vi "SMU Switch Handshaking - Debug - Continuous.vi"(8 "error in":errorcluster, 11 "file path (use dialog)":path=path "/home/lvuser/jsontestfile.json") -> (0 "error out":errorcluster)   [LabVIEW 2019]
uses:
  labview-grpc-query-server/VIs/MeasurementServer_FourProbeRawData.ctl
  labview-grpc-query-server/VIs/MeasurementServer_ErrorOutData.ctl
  JSONCluster.ctl
  <instrlib>/niDCPower/nidcpower.llb/niDCPower Send Software Edge Trigger - Signal.ctl
  <instrlib>/niDCPower/nidcpower.llb/niDCPower Wait For Event - Event.ctl
  <instrlib>/niDCPower/nidcpower.llb/niDCPower Configure Software Edge Start Trigger.vi
  <instrlib>/niDCPower/nidcpower.llb/niDCPower Configure Software Edge Sequence Advance Trigger.vi
  SupportVIs.lvlib
  labview-grpc-query-server/VIs/labview-grpc-measurement-server.lvlib
panel:
  in  "Stop":bool
  in  "Override Channel":bool
  in  "Select Next Channel":i32=39
  out "Channels Connected":string[](array[string])=["[ab0->card1r0->c39]", "[ab1->card1r1->c40]", "[ch43->com]"]
  in  "Override Settings":T1={"SMUResourceName"="SMU", "SMUChannels"="0", "SMUSourceMode"=1021, "SMUOutputFunction"=1007, "SMUSourceTransientResponse"=1038, "SMUCurrent"=1.0, "SMUCurrentLevelRange"=1.0, "SMUMeasurementSense"=1008, "SMUMeasurementApertureTime"=0.04, "SMUSourceAdvancedSourceDelay"=0.001, "SMUVoltage"=6.0, "SMUSourceAdvancedSequenceLoopCount"=162, "SMUMeasurementAdvancedDCNoiseRejection"=1044, "SMUSequenceName"="MySequence", "SMUStep1_Source_DCCurrent_CurrentLevel"=1150009, "SMUStep2_Measurement_ApertureTime"=1150058, "SMUStep3_Source_Advanced_SourceDelay"=1150051, "SMUSequenceNumberOfSteps"=3, "ScanList"="SCANALL", "Switch1ResourceName"="2526_1", "Switch1Topology"="2526/2-Wire 79x1 Mux", "Switch1ScanList"="ch70:76->com", "Switch2ResourceName"="SwitchBlock1Dev1", "Switch2Topology"="Configured Topology", "Switch2ScanList"="[c2->card1r2->c26], [c3->card1r3->c27]; [c6->card1r2->c26], [c7->card1r3->c27]; [c10->card1r2->c26], [c11->card1r3->c27]; [c14->card1r2->c26], [c15->card1r3->c27]; [c18->card1r2->c26], [c19->card1r3->c27]; [c22->card1r2->c26], [c23->card1r3->c27]; [c30->card1r2->c26], [c31->card1r3->c27];", "DMMResourceName"="DMM", "DMMFunction"=0, "DMMResolution"=0.1, "DMMRange"=0.1, "DMMSampleCount"=0, "DMMApertureTimeUnit"=0, "DMMApertureTime"=0.033, "DMMNumberOfAverages"=1, "DMMAutoZero"=0, "DMMADCCalibration"=0, "DMMSettleTime"=0.002, "DMMControlAction"=0, "DMMVoltageFaultUpperLimit"=0.0006, "ApplicationNumberOfWeldChannels"=162} {"DMMVoltageFaultUpperLimit" format="%#_6p"}
  in  "Override Settings?":bool
  out "Configured Settings":T1={"SMUResourceName"="SMU", "SMUChannels"="0", "SMUSourceMode"=1021, "SMUOutputFunction"=1007, "SMUSourceTransientResponse"=1038, "SMUCurrent"=1.0, "SMUCurrentLevelRange"=1.0, "SMUMeasurementSense"=1008, "SMUMeasurementApertureTime"=0.04, "SMUSourceAdvancedSourceDelay"=0.001, "SMUVoltage"=6.0, "SMUSourceAdvancedSequenceLoopCount"=162, "SMUMeasurementAdvancedDCNoiseRejection"=1044, "SMUSequenceName"="MySequence", "SMUStep1_Source_DCCurrent_CurrentLevel"=1150009, "SMUStep2_Measurement_ApertureTime"=1150058, "SMUStep3_Source_Advanced_SourceDelay"=1150051, "SMUSequenceNumberOfSteps"=3, "ScanList"="SCANALL", "Switch1ResourceName"="2526_1", "Switch1Topology"="2526/2-Wire 79x1 Mux", "Switch1ScanList"="ch70:76->com", "Switch2ResourceName"="SwitchBlock1Dev1", "Switch2Topology"="Configured Topology", "Switch2ScanList"="[c2->card1r2->c26], [c3->card1r3->c27]; [c6->card1r2->c26], [c7->card1r3->c27]; [c10->card1r2->c26], [c11->card1r3->c27]; [c14->card1r2->c26], [c15->card1r3->c27]; [c18->card1r2->c26], [c19->card1r3->c27]; [c22->card1r2->c26], [c23->card1r3->c27]; [c30->card1r2->c26], [c31->card1r3->c27];", "DMMResourceName"="DMM", "DMMFunction"=0, "DMMResolution"=0.1, "DMMRange"=0.1, "DMMSampleCount"=0, "DMMApertureTimeUnit"=0, "DMMApertureTime"=0.033, "DMMNumberOfAverages"=1, "DMMAutoZero"=0, "DMMADCCalibration"=0, "DMMSettleTime"=0.002, "DMMControlAction"=0, "DMMVoltageFaultUpperLimit"=0.0006, "ApplicationNumberOfWeldChannels"=162} {"DMMVoltageFaultUpperLimit" format="%#_6p"}
  out "All Results":T2[](array[typedef])=[{"Positive Voltage"=-0.05653296298856869, "Positive Current"=2.9701845245998226e-05, "Negative Voltage"=nan, "Negative Current"=3.073839441384771e-05, "Impedance"=nan, "ErrorOutData"={"ErrorCode"=-3, "ErrorMessage"="SMU HI or LO lead disconnected\n- SMU in compliance\n- SMU Fault = True\rDMM HI SENSE or LO SENSE lead disconnected\n- DMM measures NaN, or \n- DMM overrange warning, or\n- DMM voltage > 50uV "}}, {"Positive Voltage"=nan, "Positive Current"=2.9670434665157036e-05, "Negative Voltage"=nan, "Negative Current"=3.076980499469237e-05, "Impedance"=nan, "ErrorOutData"={"ErrorCode"=-3, "ErrorMessage"="SMU HI or LO lead disconnected\n- SMU in compliance\n- SMU Fault = True\rDMM HI SENSE or LO SENSE lead disconnected\n- DMM measures NaN, or \n- DMM overrange warning, or\n- DMM voltage > 50uV "}}, {"Positive Voltage"=nan, "Positive Current"=2.9796076988532205e-05, "Negative Voltage"=nan, "Negative Current"=3.070698383300305e-05, "Impedance"=nan, "ErrorOutData"={"ErrorCode"=-3, "ErrorMessage"="SMU HI or LO lead disconnected\n- SMU in compliance\n- SMU Fault = True\rDMM HI SENSE or LO SENSE lead disconnected\n- DMM measures NaN, or \n- DMM overrange warning, or\n- DMM voltage > 50uV "}}, {"Positive Voltage"=nan, "Positive Current"=2.9921719311907374e-05, "Negative Voltage"=nan, "Negative Current"=3.083262615638169e-05, "Impedance"=nan, "ErrorOutData"={"ErrorCode"=-3, "ErrorMessage"="SMU HI or LO lead disconnected\n- SMU in compliance\n- SMU Fault = True\rDMM HI SENSE or LO SENSE lead disconnected\n- DMM measures NaN, or \n- DMM overrange warning, or\n- DMM voltage > 50uV "}}, {"Positive Voltage"=nan, "Positive Current"=2.9796076988532205e-05, "Negative Voltage"=-0.04961459275744348, "Negative Current"=3.06441626713172e-05, "Impedance"=nan, "ErrorOutData"={"ErrorCode"=-3, "ErrorMessage"="SMU HI or LO lead disconnected\n- SMU in compliance\n- SMU Fault = True\rDMM HI SENSE or LO SENSE lead disconnected\n- DMM measures NaN, or \n- DMM overrange warning, or\n- DMM voltage > 50uV "}}, {"Positive Voltage"=nan, "Positive Current"=2.9858898150218055e-05, "Negative Voltage"=-0.05577502096881172, "Negative Current"=3.080121557553703e-05, "Impedance"=nan, "ErrorOutData"={"ErrorCode"=-3, "ErrorMessage"="SMU HI or LO lead disconnected\n- SMU in compliance\n- SMU Fault = True\rDMM HI SENSE or LO SENSE lead disconnected\n- DMM measures NaN, or \n- DMM overrange warning, or\n- DMM voltage > 50uV "}}, {"Positive Voltage"=0.02445423618825113, "Positive Current"=2.9890308731062715e-05, "Negative Voltage"=nan, "Negative Current"=3.09268578989122e-05, "Impedance"=nan, "ErrorOutData"={"ErrorCode"=-3, "ErrorMessage"="SMU HI or LO lead disconnected\n- SMU in compliance\n- SMU Fault = True\rDMM HI SENSE or LO SENSE lead disconnected\n- DMM measures NaN, or \n- DMM overrange warning, or\n- DMM voltage > 50uV "}}, {"Positive Voltage"=nan, "Positive Current"=2.9639024084312376e-05, "Negative Voltage"=0.01690976674095387, "Negative Current"=3.086403673722288e-05, "Impedance"=nan, "ErrorOutData"={"ErrorCode"=-3, "ErrorMessage"="SMU HI or LO lead disconnected\n- SMU in compliance\n- SMU Fault = True\rDMM HI SENSE or LO SENSE lead disconnected\n- DMM measures NaN, or \n- DMM overrange warning, or\n- DMM voltage > 50uV "}}, {"Positive Voltage"=nan, "Positive Current"=1.0000000232887618, "Negative Voltage"=-0.02788016487004771, "Negative Current"=-0.999999922774903, "Impedance"=nan, "ErrorOutData"={"ErrorCode"=-2, "ErrorMessage"="\rDMM HI SENSE or LO SENSE lead disconnected\n- DMM measures NaN, or \n- DMM overrange warning, or\n- DMM voltage > 50uV "}}, {"Positive Voltage"=nan, "Positive Current"=2.9764666407687546e-05, "Negative Voltage"=nan, "Negative Current"=3.076980499469237e-05, "Impedance"=nan, "ErrorOutData"={"ErrorCode"=-3, "ErrorMessage"="SMU HI or LO lead disconnected\n- SMU in compliance\n- SMU Fault = True\rDMM HI SENSE or LO SENSE lead disconnected\n- DMM measures NaN, or \n- DMM overrange warning, or\n- DMM voltage > 50uV "}}, {"Positive Voltage"=nan, "Positive Current"=2.9733255826842886e-05, "Negative Voltage"=nan, "Negative Current"=3.080121557553703e-05, "Impedance"=nan, "ErrorOutData"={"ErrorCode"=-3, "ErrorMessage"="SMU HI or LO lead disconnected\n- SMU in compliance\n- SMU Fault = True\rDMM HI SENSE or LO SENSE lead disconnected\n- DMM measures NaN, or \n- DMM overrange warning, or\n- DMM voltage > 50uV "}}, {"Positive Voltage"=nan, "Positive Current"=2.9764666407687546e-05, "Negative Voltage"=nan, "Negative Current"=3.070698383300305e-05, "Impedance"=nan, "ErrorOutData"={"ErrorCode"=-3, "ErrorMessage"="SMU HI or LO lead disconnected\n- SMU in compliance\n- SMU Fault = True\rDMM HI SENSE or LO SENSE lead disconnected\n- DMM measures NaN, or \n- DMM overrange warning, or\n- DMM voltage > 50uV "}}, {"Positive Voltage"=nan, "Positive Current"=2.9858898150218055e-05, "Negative Voltage"=-0.032372464954530354, "Negative Current"=3.073839441384771e-05, "Impedance"=nan, "ErrorOutData"={"ErrorCode"=-3, "ErrorMessage"="SMU HI or LO lead disconnected\n- SMU in compliance\n- SMU Fault = True\rDMM HI SENSE or LO SENSE lead disconnected\n- DMM measures NaN, or \n- DMM overrange warning, or\n- DMM voltage > 50uV "}}, {"Positive Voltage"=nan, "Positive Current"=2.9921719311907374e-05, "Negative Voltage"=nan, "Negative Current"=3.09268578989122e-05, "Impedance"=nan, "ErrorOutData"={"ErrorCode"=-3, "ErrorMessage"="SMU HI or LO lead disconnected\n- SMU in compliance\n- SMU Fault = True\rDMM HI SENSE or LO SENSE lead disconnected\n- DMM measures NaN, or \n- DMM overrange warning, or\n- DMM voltage > 50uV "}}, {"Positive Voltage"=nan, "Positive Current"=2.9858898150218055e-05, "Negative Voltage"=nan, "Negative Current"=3.0958268479756856e-05, "Impedance"=nan, "ErrorOutData"={"ErrorCode"=-3, "ErrorMessage"="SMU HI or LO lead disconnected\n- SMU in compliance\n- SMU Fault = True\rDMM HI SENSE or LO SENSE lead disconnected\n- DMM measures NaN, or \n- DMM overrange warning, or\n- DMM voltage > 50uV "}}, {"Positive Voltage"=nan, "Positive Current"=2.9764666407687546e-05, "Negative Voltage"=-0.05143121180189266, "Negative Current"=3.067557325216186e-05, "Impedance"=nan, "ErrorOutData"={"ErrorCode"=-3, "ErrorMessage"="SMU HI or LO lead disconnected\n- SMU in compliance\n- SMU Fault = True\rDMM HI SENSE or LO SENSE lead disconnected\n- DMM measures NaN, or \n- DMM overrange warning, or\n- DMM voltage > 50uV "}}, {"Positive Voltage"=nan, "Positive Current"=2.9921719311907374e-05, "Negative Voltage"=nan, "Negative Current"=3.073839441384771e-05, "Impedance"=nan, "ErrorOutData"={"ErrorCode"=-3, "ErrorMessage"="SMU HI or LO lead disconnected\n- SMU in compliance\n- SMU Fault = True\rDMM HI SENSE or LO SENSE lead disconnected\n- DMM measures NaN, or \n- DMM overrange warning, or\n- DMM voltage > 50uV "}}, {"Positive Voltage"=nan, "Positive Current"=2.9796076988532205e-05, "Negative Voltage"=nan, "Negative Current"=3.080121557553703e-05, "Impedance"=nan, "ErrorOutData"={"ErrorCode"=-3, "ErrorMessage"="SMU HI or LO lead disconnected\n- SMU in compliance\n- SMU Fault = True\rDMM HI SENSE or LO SENSE lead disconnected\n- DMM measures NaN, or \n- DMM overrange warning, or\n- DMM voltage > 50uV "}}, {"Positive Voltage"=nan, "Positive Current"=2.9764666407687546e-05, "Negative Voltage"=nan, "Negative Current"=3.089544731806754e-05, "Impedance"=nan, "ErrorOutData"={"ErrorCode"=-3, "ErrorMessage"="SMU HI or LO lead disconnected\n- SMU in compliance\n- SMU Fault = True\rDMM HI SENSE or LO SENSE lead disconnected\n- DMM measures NaN, or \n- DMM overrange warning, or\n- DMM voltage > 50uV "}}, {"Positive Voltage"=nan, "Positive Current"=2.9796076988532205e-05, "Negative Voltage"=nan, "Negative Current"=3.067557325216186e-05, "Impedance"=nan, "ErrorOutData"={"ErrorCode"=-3, "ErrorMessage"="SMU HI or LO lead disconnected\n- SMU in compliance\n- SMU Fault = True\rDMM HI SENSE or LO SENSE lead disconnected\n- DMM measures NaN, or \n- DMM overrange warning, or\n- DMM voltage > 50uV "}}, {"Positive Voltage"=nan, "Positive Current"=2.9827487569376865e-05, "Negative Voltage"=nan, "Negative Current"=3.058134150963135e-05, "Impedance"=nan, "ErrorOutData"={"ErrorCode"=-3, "ErrorMessage"="SMU HI or LO lead disconnected\n- SMU in compliance\n- SMU Fault = True\rDMM HI SENSE or LO SENSE lead disconnected\n- DMM measures NaN, or \n- DMM overrange warning, or\n- DMM voltage > 50uV "}}, {"Positive Voltage"=0.0611653266410722, "Positive Current"=2.9701845245998226e-05, "Negative Voltage"=nan, "Negative Current"=3.058134150963135e-05, "Impedance"=nan, "ErrorOutData"={"ErrorCode"=-3, "ErrorMessage"="SMU HI or LO lead disconnected\n- SMU in compliance\n- SMU Fault = True\rDMM HI SENSE or LO SENSE lead disconnected\n- DMM measures NaN, or \n- DMM overrange warning, or\n- DMM voltage > 50uV "}}, {"Positive Voltage"=nan, "Positive Current"=2.9607613503467717e-05, "Negative Voltage"=nan, "Negative Current"=3.086403673722288e-05, "Impedance"=nan, "ErrorOutData"={"ErrorCode"=-3, "ErrorMessage"="SMU HI or LO lead disconnected\n- SMU in compliance\n- SMU Fault = True\rDMM HI SENSE or LO SENSE lead disconnected\n- DMM measures NaN, or \n- DMM overrange warning, or\n- DMM voltage > 50uV "}}, {"Positive Voltage"=nan, "Positive Current"=2.9796076988532205e-05, "Negative Voltage"=nan, "Negative Current"=3.086403673722288e-05, "Impedance"=nan, "ErrorOutData"={"ErrorCode"=-3, "ErrorMessage"="SMU HI or LO lead disconnected\n- SMU in compliance\n- SMU Fault = True\rDMM HI SENSE or LO SENSE lead disconnected\n- DMM measures NaN, or \n- DMM overrange warning, or\n- DMM voltage > 50uV "}}, {"Positive Voltage"=nan, "Positive Current"=2.9670434665157036e-05, "Negative Voltage"=nan, "Negative Current"=3.06441626713172e-05, "Impedance"=nan, "ErrorOutData"={"ErrorCode"=-3, "ErrorMessage"="SMU HI or LO lead disconnected\n- SMU in compliance\n- SMU Fault = True\rDMM HI SENSE or LO SENSE lead disconnected\n- DMM measures NaN, or \n- DMM overrange warning, or\n- DMM voltage > 50uV "}}, {"Positive Voltage"=nan, "Positive Current"=2.9858898150218055e-05, "Negative Voltage"=nan, "Negative Current"=3.067557325216186e-05, "Impedance"=nan, "ErrorOutData"={"ErrorCode"=-3, "ErrorMessage"="SMU HI or LO lead disconnected\n- SMU in compliance\n- SMU Fault = True\rDMM HI SENSE or LO SENSE lead disconnected\n- DMM measures NaN, or \n- DMM overrange warning, or\n- DMM voltage > 50uV "}}, {"Positive Voltage"=nan, "Positive Current"=2.9890308731062715e-05, "Negative Voltage"=nan, "Negative Current"=3.080121557553703e-05, "Impedance"=nan, "ErrorOutData"={"ErrorCode"=-3, "ErrorMessage"="SMU HI or LO lead disconnected\n- SMU in compliance\n- SMU Fault = True\rDMM HI SENSE or LO SENSE lead disconnected\n- DMM measures NaN, or \n- DMM overrange warning, or\n- DMM voltage > 50uV "}}, {"Positive Voltage"=nan, "Positive Current"=2.9733255826842886e-05, "Negative Voltage"=nan, "Negative Current"=3.073839441384771e-05, "Impedance"=nan, "ErrorOutData"={"ErrorCode"=-3, "ErrorMessage"="SMU HI or LO lead disconnected\n- SMU in compliance\n- SMU Fault = True\rDMM HI SENSE or LO SENSE lead disconnected\n- DMM measures NaN, or \n- DMM overrange warning, or\n- DMM voltage > 50uV "}}, {"Positive Voltage"=nan, "Positive Current"=2.9670434665157036e-05, "Negative Voltage"=-0.05787915599385992, "Negative Current"=3.073839441384771e-05, "Impedance"=nan, "ErrorOutData"={"ErrorCode"=-3, "ErrorMessage"="SMU HI or LO lead disconnected\n- SMU in compliance\n- SMU Fault = True\rDMM HI SENSE or LO SENSE lead disconnected\n- DMM measures NaN, or \n- DMM overrange warning, or\n- DMM voltage > 50uV "}}, {"Positive Voltage"=nan, "Positive Current"=2.9639024084312376e-05, "Negative Voltage"=nan, "Negative Current"=3.058134150963135e-05, "Impedance"=nan, "ErrorOutData"={"ErrorCode"=-3, "ErrorMessage"="SMU HI or LO lead disconnected\n- SMU in compliance\n- SMU Fault = True\rDMM HI SENSE or LO SENSE lead disconnected\n- DMM measures NaN, or \n- DMM overrange warning, or\n- DMM voltage > 50uV "}}, {"Positive Voltage"=nan, "Positive Current"=2.9513381760937207e-05, "Negative Voltage"=nan, "Negative Current"=3.054993092878322e-05, "Impedance"=nan, "ErrorOutData"={"ErrorCode"=-3, "ErrorMessage"="SMU HI or LO lead disconnected\n- SMU in compliance\n- SMU Fault = True\rDMM HI SENSE or LO SENSE lead disconnected\n- DMM measures NaN, or \n- DMM overrange warning, or\n- DMM voltage > 50uV "}}, {"Positive Voltage"=nan, "Positive Current"=2.9670434665157036e-05, "Negative Voltage"=nan, "Negative Current"=3.061275209047254e-05, "Impedance"=nan, "ErrorOutData"={"ErrorCode"=-3, "ErrorMessage"="SMU HI or LO lead disconnected\n- SMU in compliance\n- SMU Fault = True\rDMM HI SENSE or LO SENSE lead disconnected\n- DMM measures NaN, or \n- DMM overrange warning, or\n- DMM voltage > 50uV "}}, {"Positive Voltage"=nan, "Positive Current"=2.9701845245998226e-05, "Negative Voltage"=nan, "Negative Current"=3.061275209047254e-05, "Impedance"=nan, "ErrorOutData"={"ErrorCode"=-3, "ErrorMessage"="SMU HI or LO lead disconnected\n- SMU in compliance\n- SMU Fault = True\rDMM HI SENSE or LO SENSE lead disconnected\n- DMM measures NaN, or \n- DMM overrange warning, or\n- DMM voltage > 50uV "}}, {"Positive Voltage"=nan, "Positive Current"=2.9544792341781867e-05, "Negative Voltage"=nan, "Negative Current"=3.067557325216186e-05, "Impedance"=nan, "ErrorOutData"={"ErrorCode"=-3, "ErrorMessage"="SMU HI or LO lead disconnected\n- SMU in compliance\n- SMU Fault = True\rDMM HI SENSE or LO SENSE lead disconnected\n- DMM measures NaN, or \n- DMM overrange warning, or\n- DMM voltage > 50uV "}}, {"Positive Voltage"=nan, "Positive Current"=2.9701845245998226e-05, "Negative Voltage"=nan, "Negative Current"=3.073839441384771e-05, "Impedance"=nan, "ErrorOutData"={"ErrorCode"=-3, "ErrorMessage"="SMU HI or LO lead disconnected\n- SMU in compliance\n- SMU Fault = True\rDMM HI SENSE or LO SENSE lead disconnected\n- DMM measures NaN, or \n- DMM overrange warning, or\n- DMM voltage > 50uV "}}, {"Positive Voltage"=nan, "Positive Current"=2.9513381760937207e-05, "Negative Voltage"=nan, "Negative Current"=3.06441626713172e-05, "Impedance"=nan, "ErrorOutData"={"ErrorCode"=-3, "ErrorMessage"="SMU HI or LO lead disconnected\n- SMU in compliance\n- SMU Fault = True\rDMM HI SENSE or LO SENSE lead disconnected\n- DMM measures NaN, or \n- DMM overrange warning, or\n- DMM voltage > 50uV "}}, {"Positive Voltage"=nan, "Positive Current"=2.9576202922623057e-05, "Negative Voltage"=0.0032061164902873482, "Negative Current"=3.070698383300305e-05, "Impedance"=nan, "ErrorOutData"={"ErrorCode"=-3, "ErrorMessage"="SMU HI or LO lead disconnected\n- SMU in compliance\n- SMU Fault = True\rDMM HI SENSE or LO SENSE lead disconnected\n- DMM measures NaN, or \n- DMM overrange warning, or\n- DMM voltage > 50uV "}}, {"Positive Voltage"=nan, "Positive Current"=2.9607613503467717e-05, "Negative Voltage"=-0.0014952361703153266, "Negative Current"=3.083262615638169e-05, "Impedance"=nan, "ErrorOutData"={"ErrorCode"=-3, "ErrorMessage"="SMU HI or LO lead disconnected\n- SMU in compliance\n- SMU Fault = True\rDMM HI SENSE or LO SENSE lead disconnected\n- DMM measures NaN, or \n- DMM overrange warning, or\n- DMM voltage > 50uV "}}, {"Positive Voltage"=nan, "Positive Current"=2.9796076988532205e-05, "Negative Voltage"=0.02077001908732105, "Negative Current"=3.080121557553703e-05, "Impedance"=nan, "ErrorOutData"={"ErrorCode"=-3, "ErrorMessage"="SMU HI or LO lead disconnected\n- SMU in compliance\n- SMU Fault = True\rDMM HI SENSE or LO SENSE lead disconnected\n- DMM measures NaN, or \n- DMM overrange warning, or\n- DMM voltage > 50uV "}}, {"Positive Voltage"=nan, "Positive Current"=2.9670434665157036e-05, "Negative Voltage"=0.030919103420959628, "Negative Current"=3.083262615638169e-05, "Impedance"=nan, "ErrorOutData"={"ErrorCode"=-3, "ErrorMessage"="SMU HI or LO lead disconnected\n- SMU in compliance\n- SMU Fault = True\rDMM HI SENSE or LO SENSE lead disconnected\n- DMM measures NaN, or \n- DMM overrange warning, or\n- DMM voltage > 50uV "}}, {"Positive Voltage"=nan, "Positive Current"=1.000000965606187, "Negative Voltage"=-0.057247959131579734, "Negative Current"=-1.0000000170066456, "Impedance"=nan, "ErrorOutData"={"ErrorCode"=-2, "ErrorMessage"="\rDMM HI SENSE or LO SENSE lead disconnected\n- DMM measures NaN, or \n- DMM overrange warning, or\n- DMM voltage > 50uV "}}, {"Positive Voltage"=nan, "Positive Current"=2.9576202922623057e-05, "Negative Voltage"=nan, "Negative Current"=3.06441626713172e-05, "Impedance"=nan, "ErrorOutData"={"ErrorCode"=-3, "ErrorMessage"="SMU HI or LO lead disconnected\n- SMU in compliance\n- SMU Fault = True\rDMM HI SENSE or LO SENSE lead disconnected\n- DMM measures NaN, or \n- DMM overrange warning, or\n- DMM voltage > 50uV "}}, {"Positive Voltage"=nan, "Positive Current"=2.9544792341781867e-05, "Negative Voltage"=nan, "Negative Current"=3.067557325216186e-05, "Impedance"=nan, "ErrorOutData"={"ErrorCode"=-3, "ErrorMessage"="SMU HI or LO lead disconnected\n- SMU in compliance\n- SMU Fault = True\rDMM HI SENSE or LO SENSE lead disconnected\n- DMM measures NaN, or \n- DMM overrange warning, or\n- DMM voltage > 50uV "}}, {"Positive Voltage"=nan, "Positive Current"=2.9764666407687546e-05, "Negative Voltage"=nan, "Negative Current"=3.073839441384771e-05, "Impedance"=nan, "ErrorOutData"={"ErrorCode"=-3, "ErrorMessage"="SMU HI or LO lead disconnected\n- SMU in compliance\n- SMU Fault = True\rDMM HI SENSE or LO SENSE lead disconnected\n- DMM measures NaN, or \n- DMM overrange warning, or\n- DMM voltage > 50uV "}}, {"Positive Voltage"=0.034574482900608876, "Positive Current"=2.9576202922623057e-05, "Negative Voltage"=nan, "Negative Current"=3.054993092878322e-05, "Impedance"=nan, "ErrorOutData"={"ErrorCode"=-3, "ErrorMessage"="SMU HI or LO lead disconnected\n- SMU in compliance\n- SMU Fault = True\rDMM HI SENSE or LO SENSE lead disconnected\n- DMM measures NaN, or \n- DMM overrange warning, or\n- DMM voltage > 50uV "}}, {"Positive Voltage"=nan, "Positive Current"=2.9639024084312376e-05, "Negative Voltage"=nan, "Negative Current"=3.048710976709737e-05, "Impedance"=nan, "ErrorOutData"={"ErrorCode"=-3, "ErrorMessage"="SMU HI or LO lead disconnected\n- SMU in compliance\n- SMU Fault = True\rDMM HI SENSE or LO SENSE lead disconnected\n- DMM measures NaN, or \n- DMM overrange warning, or\n- DMM voltage > 50uV "}}, {"Positive Voltage"=nan, "Positive Current"=2.9481971180092548e-05, "Negative Voltage"=nan, "Negative Current"=3.033005686287754e-05, "Impedance"=nan, "ErrorOutData"={"ErrorCode"=-3, "ErrorMessage"="SMU HI or LO lead disconnected\n- SMU in compliance\n- SMU Fault = True\rDMM HI SENSE or LO SENSE lead disconnected\n- DMM measures NaN, or \n- DMM overrange warning, or\n- DMM voltage > 50uV "}}, {"Positive Voltage"=nan, "Positive Current"=2.9387739437562038e-05, "Negative Voltage"=nan, "Negative Current"=3.03614674437222e-05, "Impedance"=nan, "ErrorOutData"={"ErrorCode"=-3, "ErrorMessage"="SMU HI or LO lead disconnected\n- SMU in compliance\n- SMU Fault = True\rDMM HI SENSE or LO SENSE lead disconnected\n- DMM measures NaN, or \n- DMM overrange warning, or\n- DMM voltage > 50uV "}}, {"Positive Voltage"=nan, "Positive Current"=2.941915001840323e-05, "Negative Voltage"=nan, "Negative Current"=3.029864628203288e-05, "Impedance"=nan, "ErrorOutData"={"ErrorCode"=-3, "ErrorMessage"="SMU HI or LO lead disconnected\n- SMU in compliance\n- SMU Fault = True\rDMM HI SENSE or LO SENSE lead disconnected\n- DMM measures NaN, or \n- DMM overrange warning, or\n- DMM voltage > 50uV "}}, {"Positive Voltage"=-0.0212574588174508, "Positive Current"=2.9387739437562038e-05, "Negative Voltage"=nan, "Negative Current"=3.03614674437222e-05, "Impedance"=nan, "ErrorOutData"={"ErrorCode"=-3, "ErrorMessage"="SMU HI or LO lead disconnected\n- SMU in compliance\n- SMU Fault = True\rDMM HI SENSE or LO SENSE lead disconnected\n- DMM measures NaN, or \n- DMM overrange warning, or\n- DMM voltage > 50uV "}}, {"Positive Voltage"=nan, "Positive Current"=2.929350769502806e-05, "Negative Voltage"=nan, "Negative Current"=3.0267235701188222e-05, "Impedance"=nan, "ErrorOutData"={"ErrorCode"=-3, "ErrorMessage"="SMU HI or LO lead disconnected\n- SMU in compliance\n- SMU Fault = True\rDMM HI SENSE or LO SENSE lead disconnected\n- DMM measures NaN, or \n- DMM overrange warning, or\n- DMM voltage > 50uV "}}, {"Positive Voltage"=nan, "Positive Current"=2.9450560599247888e-05, "Negative Voltage"=nan, "Negative Current"=3.0173003958657713e-05, "Impedance"=nan, "ErrorOutData"={"ErrorCode"=-3, "ErrorMessage"="SMU HI or LO lead disconnected\n- SMU in compliance\n- SMU Fault = True\rDMM HI SENSE or LO SENSE lead disconnected\n- DMM measures NaN, or \n- DMM overrange warning, or\n- DMM voltage > 50uV "}}, {"Positive Voltage"=0.03294451244138388, "Positive Current"=2.9576202922623057e-05, "Negative Voltage"=-0.06000793949129106, "Negative Current"=3.0204414539502372e-05, "Impedance"=-147963.59926360915, "ErrorOutData"={"ErrorCode"=-3, "ErrorMessage"="SMU HI or LO lead disconnected\n- SMU in compliance\n- SMU Fault = True\rDMM HI SENSE or LO SENSE lead disconnected\n- DMM measures NaN, or \n- DMM overrange warning, or\n- DMM voltage > 50uV "}}, {"Positive Voltage"=nan, "Positive Current"=2.935632885671738e-05, "Negative Voltage"=nan, "Negative Current"=3.03614674437222e-05, "Impedance"=nan, "ErrorOutData"={"ErrorCode"=-3, "ErrorMessage"="SMU HI or LO lead disconnected\n- SMU in compliance\n- SMU Fault = True\rDMM HI SENSE or LO SENSE lead disconnected\n- DMM measures NaN, or \n- DMM overrange warning, or\n- DMM voltage > 50uV "}}, {"Positive Voltage"=nan, "Positive Current"=2.9576202922623057e-05, "Negative Voltage"=nan, "Negative Current"=3.045569918625271e-05, "Impedance"=nan, "ErrorOutData"={"ErrorCode"=-3, "ErrorMessage"="SMU HI or LO lead disconnected\n- SMU in compliance\n- SMU Fault = True\rDMM HI SENSE or LO SENSE lead disconnected\n- DMM measures NaN, or \n- DMM overrange warning, or\n- DMM voltage > 50uV "}}, {"Positive Voltage"=nan, "Positive Current"=2.941915001840323e-05, "Negative Voltage"=nan, "Negative Current"=3.058134150963135e-05, "Impedance"=nan, "ErrorOutData"={"ErrorCode"=-3, "ErrorMessage"="SMU HI or LO lead disconnected\n- SMU in compliance\n- SMU Fault = True\rDMM HI SENSE or LO SENSE lead disconnected\n- DMM measures NaN, or \n- DMM overrange warning, or\n- DMM voltage > 50uV "}}, {"Positive Voltage"=nan, "Positive Current"=2.935632885671738e-05, "Negative Voltage"=nan, "Negative Current"=3.048710976709737e-05, "Impedance"=nan, "ErrorOutData"={"ErrorCode"=-3, "ErrorMessage"="SMU HI or LO lead disconnected\n- SMU in compliance\n- SMU Fault = True\rDMM HI SENSE or LO SENSE lead disconnected\n- DMM measures NaN, or \n- DMM overrange warning, or\n- DMM voltage > 50uV "}}, {"Positive Voltage"=nan, "Positive Current"=2.9481971180092548e-05, "Negative Voltage"=nan, "Negative Current"=3.042428860541152e-05, "Impedance"=nan, "ErrorOutData"={"ErrorCode"=-3, "ErrorMessage"="SMU HI or LO lead disconnected\n- SMU in compliance\n- SMU Fault = True\rDMM HI SENSE or LO SENSE lead disconnected\n- DMM measures NaN, or \n- DMM overrange warning, or\n- DMM voltage > 50uV "}}, {"Positive Voltage"=nan, "Positive Current"=2.9576202922623057e-05, "Negative Voltage"=nan, "Negative Current"=3.058134150963135e-05, "Impedance"=nan, "ErrorOutData"={"ErrorCode"=-3, "ErrorMessage"="SMU HI or LO lead disconnected\n- SMU in compliance\n- SMU Fault = True\rDMM HI SENSE or LO SENSE lead disconnected\n- DMM measures NaN, or \n- DMM overrange warning, or\n- DMM voltage > 50uV "}}, {"Positive Voltage"=nan, "Positive Current"=2.9796076988532205e-05, "Negative Voltage"=nan, "Negative Current"=3.061275209047254e-05, "Impedance"=nan, "ErrorOutData"={"ErrorCode"=-3, "ErrorMessage"="SMU HI or LO lead disconnected\n- SMU in compliance\n- SMU Fault = True\rDMM HI SENSE or LO SENSE lead disconnected\n- DMM measures NaN, or \n- DMM overrange warning, or\n- DMM voltage > 50uV "}}, {"Positive Voltage"=nan, "Positive Current"=2.9701845245998226e-05, "Negative Voltage"=nan, "Negative Current"=3.06441626713172e-05, "Impedance"=nan, "ErrorOutData"={"ErrorCode"=-3, "ErrorMessage"="SMU HI or LO lead disconnected\n- SMU in compliance\n- SMU Fault = True\rDMM HI SENSE or LO SENSE lead disconnected\n- DMM measures NaN, or \n- DMM overrange warning, or\n- DMM voltage > 50uV "}}, {"Positive Voltage"=nan, "Positive Current"=2.9701845245998226e-05, "Negative Voltage"=nan, "Negative Current"=3.076980499469237e-05, "Impedance"=nan, "ErrorOutData"={"ErrorCode"=-3, "ErrorMessage"="SMU HI or LO lead disconnected\n- SMU in compliance\n- SMU Fault = True\rDMM HI SENSE or LO SENSE lead disconnected\n- DMM measures NaN, or \n- DMM overrange warning, or\n- DMM voltage > 50uV "}}, {"Positive Voltage"=nan, "Positive Current"=2.9544792341781867e-05, "Negative Voltage"=nan, "Negative Current"=3.042428860541152e-05, "Impedance"=nan, "ErrorOutData"={"ErrorCode"=-3, "ErrorMessage"="SMU HI or LO lead disconnected\n- SMU in compliance\n- SMU Fault = True\rDMM HI SENSE or LO SENSE lead disconnected\n- DMM measures NaN, or \n- DMM overrange warning, or\n- DMM voltage > 50uV "}}, {"Positive Voltage"=nan, "Positive Current"=2.9639024084312376e-05, "Negative Voltage"=nan, "Negative Current"=3.058134150963135e-05, "Impedance"=nan, "ErrorOutData"={"ErrorCode"=-3, "ErrorMessage"="SMU HI or LO lead disconnected\n- SMU in compliance\n- SMU Fault = True\rDMM HI SENSE or LO SENSE lead disconnected\n- DMM measures NaN, or \n- DMM overrange warning, or\n- DMM voltage > 50uV "}}, {"Positive Voltage"=nan, "Positive Current"=2.9796076988532205e-05, "Negative Voltage"=nan, "Negative Current"=3.070698383300305e-05, "Impedance"=nan, "ErrorOutData"={"ErrorCode"=-3, "ErrorMessage"="SMU HI or LO lead disconnected\n- SMU in compliance\n- SMU Fault = True\rDMM HI SENSE or LO SENSE lead disconnected\n- DMM measures NaN, or \n- DMM overrange warning, or\n- DMM voltage > 50uV "}}, {"Positive Voltage"=nan, "Positive Current"=2.9607613503467717e-05, "Negative Voltage"=nan, "Negative Current"=3.06441626713172e-05, "Impedance"=nan, "ErrorOutData"={"ErrorCode"=-3, "ErrorMessage"="SMU HI or LO lead disconnected\n- SMU in compliance\n- SMU Fault = True\rDMM HI SENSE or LO SENSE lead disconnected\n- DMM measures NaN, or \n- DMM overrange warning, or\n- DMM voltage > 50uV "}}, {"Positive Voltage"=nan, "Positive Current"=2.9576202922623057e-05, "Negative Voltage"=nan, "Negative Current"=3.06441626713172e-05, "Impedance"=nan, "ErrorOutData"={"ErrorCode"=-3, "ErrorMessage"="SMU HI or LO lead disconnected\n- SMU in compliance\n- SMU Fault = True\rDMM HI SENSE or LO SENSE lead disconnected\n- DMM measures NaN, or \n- DMM overrange warning, or\n- DMM voltage > 50uV "}}, {"Positive Voltage"=nan, "Positive Current"=2.9513381760937207e-05, "Negative Voltage"=nan, "Negative Current"=3.058134150963135e-05, "Impedance"=nan, "ErrorOutData"={"ErrorCode"=-3, "ErrorMessage"="SMU HI or LO lead disconnected\n- SMU in compliance\n- SMU Fault = True\rDMM HI SENSE or LO SENSE lead disconnected\n- DMM measures NaN, or \n- DMM overrange warning, or\n- DMM voltage > 50uV "}}, {"Positive Voltage"=nan, "Positive Current"=2.9576202922623057e-05, "Negative Voltage"=nan, "Negative Current"=3.051852034794203e-05, "Impedance"=nan, "ErrorOutData"={"ErrorCode"=-3, "ErrorMessage"="SMU HI or LO lead disconnected\n- SMU in compliance\n- SMU Fault = True\rDMM HI SENSE or LO SENSE lead disconnected\n- DMM measures NaN, or \n- DMM overrange warning, or\n- DMM voltage > 50uV "}}, {"Positive Voltage"=-0.0305689879447921, "Positive Current"=2.9670434665157036e-05, "Negative Voltage"=0.035390038606321006, "Negative Current"=3.067557325216186e-05, "Impedance"=65621.82310367978, "ErrorOutData"={"ErrorCode"=-1, "ErrorMessage"="SMU HI or LO lead disconnected\n- SMU in compliance\n- SMU Fault = True\r"}}, {"Positive Voltage"=nan, "Positive Current"=2.9701845245998226e-05, "Negative Voltage"=nan, "Negative Current"=3.042428860541152e-05, "Impedance"=nan, "ErrorOutData"={"ErrorCode"=-3, "ErrorMessage"="SMU HI or LO lead disconnected\n- SMU in compliance\n- SMU Fault = True\rDMM HI SENSE or LO SENSE lead disconnected\n- DMM measures NaN, or \n- DMM overrange warning, or\n- DMM voltage > 50uV "}}, {"Positive Voltage"=0.04159997666512517, "Positive Current"=2.941915001840323e-05, "Negative Voltage"=-0.021311611621380643, "Negative Current"=3.058134150963135e-05, "Impedance"=-54131.86102406012, "ErrorOutData"={"ErrorCode"=-3, "ErrorMessage"="SMU HI or LO lead disconnected\n- SMU in compliance\n- SMU Fault = True\rDMM HI SENSE or LO SENSE lead disconnected\n- DMM measures NaN, or \n- DMM overrange warning, or\n- DMM voltage > 50uV "}}, {"Positive Voltage"=nan, "Positive Current"=2.9481971180092548e-05, "Negative Voltage"=nan, "Negative Current"=3.06441626713172e-05, "Impedance"=nan, "ErrorOutData"={"ErrorCode"=-3, "ErrorMessage"="SMU HI or LO lead disconnected\n- SMU in compliance\n- SMU Fault = True\rDMM HI SENSE or LO SENSE lead disconnected\n- DMM measures NaN, or \n- DMM overrange warning, or\n- DMM voltage > 50uV "}}, {"Positive Voltage"=nan, "Positive Current"=2.9607613503467717e-05, "Negative Voltage"=-0.053258379557544575, "Negative Current"=3.06441626713172e-05, "Impedance"=nan, "ErrorOutData"={"ErrorCode"=-3, "ErrorMessage"="SMU HI or LO lead disconnected\n- SMU in compliance\n- SMU Fault = True\rDMM HI SENSE or LO SENSE lead disconnected\n- DMM measures NaN, or \n- DMM overrange warning, or\n- DMM voltage > 50uV "}}, {"Positive Voltage"=nan, "Positive Current"=2.9670434665157036e-05, "Negative Voltage"=nan, "Negative Current"=3.058134150963135e-05, "Impedance"=nan, "ErrorOutData"={"ErrorCode"=-3, "ErrorMessage"="SMU HI or LO lead disconnected\n- SMU in compliance\n- SMU Fault = True\rDMM HI SENSE or LO SENSE lead disconnected\n- DMM measures NaN, or \n- DMM overrange warning, or\n- DMM voltage > 50uV "}}, {"Positive Voltage"=nan, "Positive Current"=2.9701845245998226e-05, "Negative Voltage"=0.04240172396042548, "Negative Current"=3.067557325216186e-05, "Impedance"=nan, "ErrorOutData"={"ErrorCode"=-3, "ErrorMessage"="SMU HI or LO lead disconnected\n- SMU in compliance\n- SMU Fault = True\rDMM HI SENSE or LO SENSE lead disconnected\n- DMM measures NaN, or \n- DMM overrange warning, or\n- DMM voltage > 50uV "}}, {"Positive Voltage"=nan, "Positive Current"=2.9670434665157036e-05, "Negative Voltage"=nan, "Negative Current"=3.058134150963135e-05, "Impedance"=nan, "ErrorOutData"={"ErrorCode"=-3, "ErrorMessage"="SMU HI or LO lead disconnected\n- SMU in compliance\n- SMU Fault = True\rDMM HI SENSE or LO SENSE lead disconnected\n- DMM measures NaN, or \n- DMM overrange warning, or\n- DMM voltage > 50uV "}}, {"Positive Voltage"=nan, "Positive Current"=2.9639024084312376e-05, "Negative Voltage"=nan, "Negative Current"=3.067557325216186e-05, "Impedance"=nan, "ErrorOutData"={"ErrorCode"=-3, "ErrorMessage"="SMU HI or LO lead disconnected\n- SMU in compliance\n- SMU Fault = True\rDMM HI SENSE or LO SENSE lead disconnected\n- DMM measures NaN, or \n- DMM overrange warning, or\n- DMM voltage > 50uV "}}, {"Positive Voltage"=nan, "Positive Current"=2.9701845245998226e-05, "Negative Voltage"=nan, "Negative Current"=3.076980499469237e-05, "Impedance"=nan, "ErrorOutData"={"ErrorCode"=-3, "ErrorMessage"="SMU HI or LO lead disconnected\n- SMU in compliance\n- SMU Fault = True\rDMM HI SENSE or LO SENSE lead disconnected\n- DMM measures NaN, or \n- DMM overrange warning, or\n- DMM voltage > 50uV "}}, {"Positive Voltage"=nan, "Positive Current"=2.9796076988532205e-05, "Negative Voltage"=nan, "Negative Current"=3.070698383300305e-05, "Impedance"=nan, "ErrorOutData"={"ErrorCode"=-3, "ErrorMessage"="SMU HI or LO lead disconnected\n- SMU in compliance\n- SMU Fault = True\rDMM HI SENSE or LO SENSE lead disconnected\n- DMM measures NaN, or \n- DMM overrange warning, or\n- DMM voltage > 50uV "}}, {"Positive Voltage"=nan, "Positive Current"=2.9701845245998226e-05, "Negative Voltage"=0.01155661965416269, "Negative Current"=3.061275209047254e-05, "Impedance"=nan, "ErrorOutData"={"ErrorCode"=-3, "ErrorMessage"="SMU HI or LO lead disconnected\n- SMU in compliance\n- SMU Fault = True\rDMM HI SENSE or LO SENSE lead disconnected\n- DMM measures NaN, or \n- DMM overrange warning, or\n- DMM voltage > 50uV "}}, {"Positive Voltage"=nan, "Positive Current"=2.9670434665157036e-05, "Negative Voltage"=nan, "Negative Current"=3.054993092878322e-05, "Impedance"=nan, "ErrorOutData"={"ErrorCode"=-3, "ErrorMessage"="SMU HI or LO lead disconnected\n- SMU in compliance\n- SMU Fault = True\rDMM HI SENSE or LO SENSE lead disconnected\n- DMM measures NaN, or \n- DMM overrange warning, or\n- DMM voltage > 50uV "}}, {"Positive Voltage"=nan, "Positive Current"=2.9701845245998226e-05, "Negative Voltage"=-0.01666067758274105, "Negative Current"=3.070698383300305e-05, "Impedance"=nan, "ErrorOutData"={"ErrorCode"=-3, "ErrorMessage"="SMU HI or LO lead disconnected\n- SMU in compliance\n- SMU Fault = True\rDMM HI SENSE or LO SENSE lead disconnected\n- DMM measures NaN, or \n- DMM overrange warning, or\n- DMM voltage > 50uV "}}, {"Positive Voltage"=nan, "Positive Current"=2.9576202922623057e-05, "Negative Voltage"=nan, "Negative Current"=3.06441626713172e-05, "Impedance"=nan, "ErrorOutData"={"ErrorCode"=-3, "ErrorMessage"="SMU HI or LO lead disconnected\n- SMU in compliance\n- SMU Fault = True\rDMM HI SENSE or LO SENSE lead disconnected\n- DMM measures NaN, or \n- DMM overrange warning, or\n- DMM voltage > 50uV "}}, {"Positive Voltage"=nan, "Positive Current"=2.9513381760937207e-05, "Negative Voltage"=nan, "Negative Current"=3.073839441384771e-05, "Impedance"=nan, "ErrorOutData"={"ErrorCode"=-3, "ErrorMessage"="SMU HI or LO lead disconnected\n- SMU in compliance\n- SMU Fault = True\rDMM HI SENSE or LO SENSE lead disconnected\n- DMM measures NaN, or \n- DMM overrange warning, or\n- DMM voltage > 50uV "}}, {"Positive Voltage"=nan, "Positive Current"=2.9607613503467717e-05, "Negative Voltage"=nan, "Negative Current"=3.058134150963135e-05, "Impedance"=nan, "ErrorOutData"={"ErrorCode"=-3, "ErrorMessage"="SMU HI or LO lead disconnected\n- SMU in compliance\n- SMU Fault = True\rDMM HI SENSE or LO SENSE lead disconnected\n- DMM measures NaN, or \n- DMM overrange warning, or\n- DMM voltage > 50uV "}}, {"Positive Voltage"=nan, "Positive Current"=2.9670434665157036e-05, "Negative Voltage"=nan, "Negative Current"=3.045569918625271e-05, "Impedance"=nan, "ErrorOutData"={"ErrorCode"=-3, "ErrorMessage"="SMU HI or LO lead disconnected\n- SMU in compliance\n- SMU Fault = True\rDMM HI SENSE or LO SENSE lead disconnected\n- DMM measures NaN, or \n- DMM overrange warning, or\n- DMM voltage > 50uV "}}, {"Positive Voltage"=nan, "Positive Current"=2.9576202922623057e-05, "Negative Voltage"=nan, "Negative Current"=3.054993092878322e-05, "Impedance"=nan, "ErrorOutData"={"ErrorCode"=-3, "ErrorMessage"="SMU HI or LO lead disconnected\n- SMU in compliance\n- SMU Fault = True\rDMM HI SENSE or LO SENSE lead disconnected\n- DMM measures NaN, or \n- DMM overrange warning, or\n- DMM voltage > 50uV "}}, {"Positive Voltage"=nan, "Positive Current"=2.9607613503467717e-05, "Negative Voltage"=nan, "Negative Current"=3.070698383300305e-05, "Impedance"=nan, "ErrorOutData"={"ErrorCode"=-3, "ErrorMessage"="SMU HI or LO lead disconnected\n- SMU in compliance\n- SMU Fault = True\rDMM HI SENSE or LO SENSE lead disconnected\n- DMM measures NaN, or \n- DMM overrange warning, or\n- DMM voltage > 50uV "}}, {"Positive Voltage"=nan, "Positive Current"=2.9513381760937207e-05, "Negative Voltage"=nan, "Negative Current"=3.048710976709737e-05, "Impedance"=nan, "ErrorOutData"={"ErrorCode"=-3, "ErrorMessage"="SMU HI or LO lead disconnected\n- SMU in compliance\n- SMU Fault = True\rDMM HI SENSE or LO SENSE lead disconnected\n- DMM measures NaN, or \n- DMM overrange warning, or\n- DMM voltage > 50uV "}}, {"Positive Voltage"=nan, "Positive Current"=2.9513381760937207e-05, "Negative Voltage"=nan, "Negative Current"=3.054993092878322e-05, "Impedance"=nan, "ErrorOutData"={"ErrorCode"=-3, "ErrorMessage"="SMU HI or LO lead disconnected\n- SMU in compliance\n- SMU Fault = True\rDMM HI SENSE or LO SENSE lead disconnected\n- DMM measures NaN, or \n- DMM overrange warning, or\n- DMM voltage > 50uV "}}, {"Positive Voltage"=nan, "Positive Current"=2.9481971180092548e-05, "Negative Voltage"=0.03870498940037781, "Negative Current"=3.03614674437222e-05, "Impedance"=nan, "ErrorOutData"={"ErrorCode"=-3, "ErrorMessage"="SMU HI or LO lead disconnected\n- SMU in compliance\n- SMU Fault = True\rDMM HI SENSE or LO SENSE lead disconnected\n- DMM measures NaN, or \n- DMM overrange warning, or\n- DMM voltage > 50uV "}}, {"Positive Voltage"=nan, "Positive Current"=2.9450560599247888e-05, "Negative Voltage"=0.051067666628266783, "Negative Current"=3.048710976709737e-05, "Impedance"=nan, "ErrorOutData"={"ErrorCode"=-3, "ErrorMessage"="SMU HI or LO lead disconnected\n- SMU in compliance\n- SMU Fault = True\rDMM HI SENSE or LO SENSE lead disconnected\n- DMM measures NaN, or \n- DMM overrange warning, or\n- DMM voltage > 50uV "}}, {"Positive Voltage"=nan, "Positive Current"=0.9999998976464385, "Negative Voltage"=nan, "Negative Current"=-0.999999922774903, "Impedance"=nan, "ErrorOutData"={"ErrorCode"=-2, "ErrorMessage"="\rDMM HI SENSE or LO SENSE lead disconnected\n- DMM measures NaN, or \n- DMM overrange warning, or\n- DMM voltage > 50uV "}}, {"Positive Voltage"=nan, "Positive Current"=2.932491827587272e-05, "Negative Voltage"=nan, "Negative Current"=3.033005686287754e-05, "Impedance"=nan, "ErrorOutData"={"ErrorCode"=-3, "ErrorMessage"="SMU HI or LO lead disconnected\n- SMU in compliance\n- SMU Fault = True\rDMM HI SENSE or LO SENSE lead disconnected\n- DMM measures NaN, or \n- DMM overrange warning, or\n- DMM voltage > 50uV "}}, {"Positive Voltage"=nan, "Positive Current"=2.9450560599247888e-05, "Negative Voltage"=nan, "Negative Current"=3.054993092878322e-05, "Impedance"=nan, "ErrorOutData"={"ErrorCode"=-3, "ErrorMessage"="SMU HI or LO lead disconnected\n- SMU in compliance\n- SMU Fault = True\rDMM HI SENSE or LO SENSE lead disconnected\n- DMM measures NaN, or \n- DMM overrange warning, or\n- DMM voltage > 50uV "}}, {"Positive Voltage"=nan, "Positive Current"=2.9450560599247888e-05, "Negative Voltage"=nan, "Negative Current"=3.051852034794203e-05, "Impedance"=nan, "ErrorOutData"={"ErrorCode"=-3, "ErrorMessage"="SMU HI or LO lead disconnected\n- SMU in compliance\n- SMU Fault = True\rDMM HI SENSE or LO SENSE lead disconnected\n- DMM measures NaN, or \n- DMM overrange warning, or\n- DMM voltage > 50uV "}}, {"Positive Voltage"=nan, "Positive Current"=2.9701845245998226e-05, "Negative Voltage"=-0.05054200197056223, "Negative Current"=3.042428860541152e-05, "Impedance"=nan, "ErrorOutData"={"ErrorCode"=-3, "ErrorMessage"="SMU HI or LO lead disconnected\n- SMU in compliance\n- SMU Fault = True\rDMM HI SENSE or LO SENSE lead disconnected\n- DMM measures NaN, or \n- DMM overrange warning, or\n- DMM voltage > 50uV "}}, {"Positive Voltage"=nan, "Positive Current"=2.941915001840323e-05, "Negative Voltage"=nan, "Negative Current"=3.045569918625271e-05, "Impedance"=nan, "ErrorOutData"={"ErrorCode"=-3, "ErrorMessage"="SMU HI or LO lead disconnected\n- SMU in compliance\n- SMU Fault = True\rDMM HI SENSE or LO SENSE lead disconnected\n- DMM measures NaN, or \n- DMM overrange warning, or\n- DMM voltage > 50uV "}}, {"Positive Voltage"=nan, "Positive Current"=2.9450560599247888e-05, "Negative Voltage"=-0.05516843099421177, "Negative Current"=3.0267235701188222e-05, "Impedance"=nan, "ErrorOutData"={"ErrorCode"=-3, "ErrorMessage"="SMU HI or LO lead disconnected\n- SMU in compliance\n- SMU Fault = True\rDMM HI SENSE or LO SENSE lead disconnected\n- DMM measures NaN, or \n- DMM overrange warning, or\n- DMM voltage > 50uV "}}, {"Positive Voltage"=nan, "Positive Current"=2.9576202922623057e-05, "Negative Voltage"=nan, "Negative Current"=3.042428860541152e-05, "Impedance"=nan, "ErrorOutData"={"ErrorCode"=-3, "ErrorMessage"="SMU HI or LO lead disconnected\n- SMU in compliance\n- SMU Fault = True\rDMM HI SENSE or LO SENSE lead disconnected\n- DMM measures NaN, or \n- DMM overrange warning, or\n- DMM voltage > 50uV "}}, {"Positive Voltage"=nan, "Positive Current"=2.9481971180092548e-05, "Negative Voltage"=nan, "Negative Current"=3.029864628203288e-05, "Impedance"=nan, "ErrorOutData"={"ErrorCode"=-3, "ErrorMessage"="SMU HI or LO lead disconnected\n- SMU in compliance\n- SMU Fault = True\rDMM HI SENSE or LO SENSE lead disconnected\n- DMM measures NaN, or \n- DMM overrange warning, or\n- DMM voltage > 50uV "}}, {"Positive Voltage"=nan, "Positive Current"=2.935632885671738e-05, "Negative Voltage"=nan, "Negative Current"=3.033005686287754e-05, "Impedance"=nan, "ErrorOutData"={"ErrorCode"=-3, "ErrorMessage"="SMU HI or LO lead disconnected\n- SMU in compliance\n- SMU Fault = True\rDMM HI SENSE or LO SENSE lead disconnected\n- DMM measures NaN, or \n- DMM overrange warning, or\n- DMM voltage > 50uV "}}, {"Positive Voltage"=nan, "Positive Current"=2.9481971180092548e-05, "Negative Voltage"=nan, "Negative Current"=3.045569918625271e-05, "Impedance"=nan, "ErrorOutData"={"ErrorCode"=-3, "ErrorMessage"="SMU HI or LO lead disconnected\n- SMU in compliance\n- SMU Fault = True\rDMM HI SENSE or LO SENSE lead disconnected\n- DMM measures NaN, or \n- DMM overrange warning, or\n- DMM voltage > 50uV "}}, {"Positive Voltage"=nan, "Positive Current"=2.9450560599247888e-05, "Negative Voltage"=nan, "Negative Current"=3.03614674437222e-05, "Impedance"=nan, "ErrorOutData"={"ErrorCode"=-3, "ErrorMessage"="SMU HI or LO lead disconnected\n- SMU in compliance\n- SMU Fault = True\rDMM HI SENSE or LO SENSE lead disconnected\n- DMM measures NaN, or \n- DMM overrange warning, or\n- DMM voltage > 50uV "}}, {"Positive Voltage"=nan, "Positive Current"=2.9450560599247888e-05, "Negative Voltage"=-0.02266117833381058, "Negative Current"=3.051852034794203e-05, "Impedance"=nan, "ErrorOutData"={"ErrorCode"=-3, "ErrorMessage"="SMU HI or LO lead disconnected\n- SMU in compliance\n- SMU Fault = True\rDMM HI SENSE or LO SENSE lead disconnected\n- DMM measures NaN, or \n- DMM overrange warning, or\n- DMM voltage > 50uV "}}, {"Positive Voltage"=nan, "Positive Current"=2.9481971180092548e-05, "Negative Voltage"=nan, "Negative Current"=3.039287802456686e-05, "Impedance"=nan, "ErrorOutData"={"ErrorCode"=-3, "ErrorMessage"="SMU HI or LO lead disconnected\n- SMU in compliance\n- SMU Fault = True\rDMM HI SENSE or LO SENSE lead disconnected\n- DMM measures NaN, or \n- DMM overrange warning, or\n- DMM voltage > 50uV "}}, {"Positive Voltage"=nan, "Positive Current"=2.9544792341781867e-05, "Negative Voltage"=nan, "Negative Current"=3.03614674437222e-05, "Impedance"=nan, "ErrorOutData"={"ErrorCode"=-3, "ErrorMessage"="SMU HI or LO lead disconnected\n- SMU in compliance\n- SMU Fault = True\rDMM HI SENSE or LO SENSE lead disconnected\n- DMM measures NaN, or \n- DMM overrange warning, or\n- DMM voltage > 50uV "}}, {"Positive Voltage"=0.025701832670473358, "Positive Current"=2.9513381760937207e-05, "Negative Voltage"=nan, "Negative Current"=3.051852034794203e-05, "Impedance"=nan, "ErrorOutData"={"ErrorCode"=-3, "ErrorMessage"="SMU HI or LO lead disconnected\n- SMU in compliance\n- SMU Fault = True\rDMM HI SENSE or LO SENSE lead disconnected\n- DMM measures NaN, or \n- DMM overrange warning, or\n- DMM voltage > 50uV "}}, {"Positive Voltage"=nan, "Positive Current"=2.9576202922623057e-05, "Negative Voltage"=nan, "Negative Current"=3.048710976709737e-05, "Impedance"=nan, "ErrorOutData"={"ErrorCode"=-3, "ErrorMessage"="SMU HI or LO lead disconnected\n- SMU in compliance\n- SMU Fault = True\rDMM HI SENSE or LO SENSE lead disconnected\n- DMM measures NaN, or \n- DMM overrange warning, or\n- DMM voltage > 50uV "}}, {"Positive Voltage"=nan, "Positive Current"=2.9387739437562038e-05, "Negative Voltage"=nan, "Negative Current"=3.039287802456686e-05, "Impedance"=nan, "ErrorOutData"={"ErrorCode"=-3, "ErrorMessage"="SMU HI or LO lead disconnected\n- SMU in compliance\n- SMU Fault = True\rDMM HI SENSE or LO SENSE lead disconnected\n- DMM measures NaN, or \n- DMM overrange warning, or\n- DMM voltage > 50uV "}}, {"Positive Voltage"=nan, "Positive Current"=2.9607613503467717e-05, "Negative Voltage"=nan, "Negative Current"=3.048710976709737e-05, "Impedance"=nan, "ErrorOutData"={"ErrorCode"=-3, "ErrorMessage"="SMU HI or LO lead disconnected\n- SMU in compliance\n- SMU Fault = True\rDMM HI SENSE or LO SENSE lead disconnected\n- DMM measures NaN, or \n- DMM overrange warning, or\n- DMM voltage > 50uV "}}, {"Positive Voltage"=nan, "Positive Current"=2.932491827587272e-05, "Negative Voltage"=nan, "Negative Current"=3.042428860541152e-05, "Impedance"=nan, "ErrorOutData"={"ErrorCode"=-3, "ErrorMessage"="SMU HI or LO lead disconnected\n- SMU in compliance\n- SMU Fault = True\rDMM HI SENSE or LO SENSE lead disconnected\n- DMM measures NaN, or \n- DMM overrange warning, or\n- DMM voltage > 50uV "}}, {"Positive Voltage"=nan, "Positive Current"=2.9481971180092548e-05, "Negative Voltage"=-0.056757794106663664, "Negative Current"=3.054993092878322e-05, "Impedance"=nan, "ErrorOutData"={"ErrorCode"=-3, "ErrorMessage"="SMU HI or LO lead disconnected\n- SMU in compliance\n- SMU Fault = True\rDMM HI SENSE or LO SENSE lead disconnected\n- DMM measures NaN, or \n- DMM overrange warning, or\n- DMM voltage > 50uV "}}, {"Positive Voltage"=nan, "Positive Current"=2.935632885671738e-05, "Negative Voltage"=nan, "Negative Current"=3.048710976709737e-05, "Impedance"=nan, "ErrorOutData"={"ErrorCode"=-3, "ErrorMessage"="SMU HI or LO lead disconnected\n- SMU in compliance\n- SMU Fault = True\rDMM HI SENSE or LO SENSE lead disconnected\n- DMM measures NaN, or \n- DMM overrange warning, or\n- DMM voltage > 50uV "}}, {"Positive Voltage"=nan, "Positive Current"=2.941915001840323e-05, "Negative Voltage"=nan, "Negative Current"=3.033005686287754e-05, "Impedance"=nan, "ErrorOutData"={"ErrorCode"=-3, "ErrorMessage"="SMU HI or LO lead disconnected\n- SMU in compliance\n- SMU Fault = True\rDMM HI SENSE or LO SENSE lead disconnected\n- DMM measures NaN, or \n- DMM overrange warning, or\n- DMM voltage > 50uV "}}, {"Positive Voltage"=nan, "Positive Current"=2.9387739437562038e-05, "Negative Voltage"=nan, "Negative Current"=3.03614674437222e-05, "Impedance"=nan, "ErrorOutData"={"ErrorCode"=-3, "ErrorMessage"="SMU HI or LO lead disconnected\n- SMU in compliance\n- SMU Fault = True\rDMM HI SENSE or LO SENSE lead disconnected\n- DMM measures NaN, or \n- DMM overrange warning, or\n- DMM voltage > 50uV "}}, {"Positive Voltage"=nan, "Positive Current"=2.9387739437562038e-05, "Negative Voltage"=nan, "Negative Current"=3.039287802456686e-05, "Impedance"=nan, "ErrorOutData"={"ErrorCode"=-3, "ErrorMessage"="SMU HI or LO lead disconnected\n- SMU in compliance\n- SMU Fault = True\rDMM HI SENSE or LO SENSE lead disconnected\n- DMM measures NaN, or \n- DMM overrange warning, or\n- DMM voltage > 50uV "}}, {"Positive Voltage"=nan, "Positive Current"=2.935632885671738e-05, "Negative Voltage"=nan, "Negative Current"=3.051852034794203e-05, "Impedance"=nan, "ErrorOutData"={"ErrorCode"=-3, "ErrorMessage"="SMU HI or LO lead disconnected\n- SMU in compliance\n- SMU Fault = True\rDMM HI SENSE or LO SENSE lead disconnected\n- DMM measures NaN, or \n- DMM overrange warning, or\n- DMM voltage > 50uV "}}, {"Positive Voltage"=nan, "Positive Current"=2.9607613503467717e-05, "Negative Voltage"=nan, "Negative Current"=3.048710976709737e-05, "Impedance"=nan, "ErrorOutData"={"ErrorCode"=-3, "ErrorMessage"="SMU HI or LO lead disconnected\n- SMU in compliance\n- SMU Fault = True\rDMM HI SENSE or LO SENSE lead disconnected\n- DMM measures NaN, or \n- DMM overrange warning, or\n- DMM voltage > 50uV "}}, {"Positive Voltage"=nan, "Positive Current"=2.9607613503467717e-05, "Negative Voltage"=nan, "Negative Current"=3.042428860541152e-05, "Impedance"=nan, "ErrorOutData"={"ErrorCode"=-3, "ErrorMessage"="SMU HI or LO lead disconnected\n- SMU in compliance\n- SMU Fault = True\rDMM HI SENSE or LO SENSE lead disconnected\n- DMM measures NaN, or \n- DMM overrange warning, or\n- DMM voltage > 50uV "}}, {"Positive Voltage"=nan, "Positive Current"=2.9450560599247888e-05, "Negative Voltage"=nan, "Negative Current"=3.033005686287754e-05, "Impedance"=nan, "ErrorOutData"={"ErrorCode"=-3, "ErrorMessage"="SMU HI or LO lead disconnected\n- SMU in compliance\n- SMU Fault = True\rDMM HI SENSE or LO SENSE lead disconnected\n- DMM measures NaN, or \n- DMM overrange warning, or\n- DMM voltage > 50uV "}}, {"Positive Voltage"=0.03039337383928046, "Positive Current"=2.9450560599247888e-05, "Negative Voltage"=nan, "Negative Current"=3.03614674437222e-05, "Impedance"=nan, "ErrorOutData"={"ErrorCode"=-3, "ErrorMessage"="SMU HI or LO lead disconnected\n- SMU in compliance\n- SMU Fault = True\rDMM HI SENSE or LO SENSE lead disconnected\n- DMM measures NaN, or \n- DMM overrange warning, or\n- DMM voltage > 50uV "}}, {"Positive Voltage"=nan, "Positive Current"=2.935632885671738e-05, "Negative Voltage"=nan, "Negative Current"=3.042428860541152e-05, "Impedance"=nan, "ErrorOutData"={"ErrorCode"=-3, "ErrorMessage"="SMU HI or LO lead disconnected\n- SMU in compliance\n- SMU Fault = True\rDMM HI SENSE or LO SENSE lead disconnected\n- DMM measures NaN, or \n- DMM overrange warning, or\n- DMM voltage > 50uV "}}, {"Positive Voltage"=nan, "Positive Current"=2.9513381760937207e-05, "Negative Voltage"=nan, "Negative Current"=3.048710976709737e-05, "Impedance"=nan, "ErrorOutData"={"ErrorCode"=-3, "ErrorMessage"="SMU HI or LO lead disconnected\n- SMU in compliance\n- SMU Fault = True\rDMM HI SENSE or LO SENSE lead disconnected\n- DMM measures NaN, or \n- DMM overrange warning, or\n- DMM voltage > 50uV "}}, {"Positive Voltage"=nan, "Positive Current"=2.941915001840323e-05, "Negative Voltage"=nan, "Negative Current"=3.048710976709737e-05, "Impedance"=nan, "ErrorOutData"={"ErrorCode"=-3, "ErrorMessage"="SMU HI or LO lead disconnected\n- SMU in compliance\n- SMU Fault = True\rDMM HI SENSE or LO SENSE lead disconnected\n- DMM measures NaN, or \n- DMM overrange warning, or\n- DMM voltage > 50uV "}}, {"Positive Voltage"=0.018763033638299988, "Positive Current"=2.9481971180092548e-05, "Negative Voltage"=nan, "Negative Current"=3.029864628203288e-05, "Impedance"=nan, "ErrorOutData"={"ErrorCode"=-3, "ErrorMessage"="SMU HI or LO lead disconnected\n- SMU in compliance\n- SMU Fault = True\rDMM HI SENSE or LO SENSE lead disconnected\n- DMM measures NaN, or \n- DMM overrange warning, or\n- DMM voltage > 50uV "}}, {"Positive Voltage"=nan, "Positive Current"=2.9450560599247888e-05, "Negative Voltage"=nan, "Negative Current"=3.045569918625271e-05, "Impedance"=nan, "ErrorOutData"={"ErrorCode"=-3, "ErrorMessage"="SMU HI or LO lead disconnected\n- SMU in compliance\n- SMU Fault = True\rDMM HI SENSE or LO SENSE lead disconnected\n- DMM measures NaN, or \n- DMM overrange warning, or\n- DMM voltage > 50uV "}}, {"Positive Voltage"=nan, "Positive Current"=2.929350769502806e-05, "Negative Voltage"=nan, "Negative Current"=3.0204414539502372e-05, "Impedance"=nan, "ErrorOutData"={"ErrorCode"=-3, "ErrorMessage"="SMU HI or LO lead disconnected\n- SMU in compliance\n- SMU Fault = True\rDMM HI SENSE or LO SENSE lead disconnected\n- DMM measures NaN, or \n- DMM overrange warning, or\n- DMM voltage > 50uV "}}, {"Positive Voltage"=nan, "Positive Current"=2.9387739437562038e-05, "Negative Voltage"=nan, "Negative Current"=3.042428860541152e-05, "Impedance"=nan, "ErrorOutData"={"ErrorCode"=-3, "ErrorMessage"="SMU HI or LO lead disconnected\n- SMU in compliance\n- SMU Fault = True\rDMM HI SENSE or LO SENSE lead disconnected\n- DMM measures NaN, or \n- DMM overrange warning, or\n- DMM voltage > 50uV "}}, {"Positive Voltage"=nan, "Positive Current"=2.941915001840323e-05, "Negative Voltage"=nan, "Negative Current"=3.03614674437222e-05, "Impedance"=nan, "ErrorOutData"={"ErrorCode"=-3, "ErrorMessage"="SMU HI or LO lead disconnected\n- SMU in compliance\n- SMU Fault = True\rDMM HI SENSE or LO SENSE lead disconnected\n- DMM measures NaN, or \n- DMM overrange warning, or\n- DMM voltage > 50uV "}}, {"Positive Voltage"=nan, "Positive Current"=2.9450560599247888e-05, "Negative Voltage"=nan, "Negative Current"=3.042428860541152e-05, "Impedance"=nan, "ErrorOutData"={"ErrorCode"=-3, "ErrorMessage"="SMU HI or LO lead disconnected\n- SMU in compliance\n- SMU Fault = True\rDMM HI SENSE or LO SENSE lead disconnected\n- DMM measures NaN, or \n- DMM overrange warning, or\n- DMM voltage > 50uV "}}, {"Positive Voltage"=nan, "Positive Current"=2.9481971180092548e-05, "Negative Voltage"=nan, "Negative Current"=3.051852034794203e-05, "Impedance"=nan, "ErrorOutData"={"ErrorCode"=-3, "ErrorMessage"="SMU HI or LO lead disconnected\n- SMU in compliance\n- SMU Fault = True\rDMM HI SENSE or LO SENSE lead disconnected\n- DMM measures NaN, or \n- DMM overrange warning, or\n- DMM voltage > 50uV "}}, {"Positive Voltage"=nan, "Positive Current"=2.9387739437562038e-05, "Negative Voltage"=nan, "Negative Current"=3.054993092878322e-05, "Impedance"=nan, "ErrorOutData"={"ErrorCode"=-3, "ErrorMessage"="SMU HI or LO lead disconnected\n- SMU in compliance\n- SMU Fault = True\rDMM HI SENSE or LO SENSE lead disconnected\n- DMM measures NaN, or \n- DMM overrange warning, or\n- DMM voltage > 50uV "}}, {"Positive Voltage"=nan, "Positive Current"=2.9576202922623057e-05, "Negative Voltage"=nan, "Negative Current"=3.054993092878322e-05, "Impedance"=nan, "ErrorOutData"={"ErrorCode"=-3, "ErrorMessage"="SMU HI or LO lead disconnected\n- SMU in compliance\n- SMU Fault = True\rDMM HI SENSE or LO SENSE lead disconnected\n- DMM measures NaN, or \n- DMM overrange warning, or\n- DMM voltage > 50uV "}}, {"Positive Voltage"=nan, "Positive Current"=2.9576202922623057e-05, "Negative Voltage"=nan, "Negative Current"=3.039287802456686e-05, "Impedance"=nan, "ErrorOutData"={"ErrorCode"=-3, "ErrorMessage"="SMU HI or LO lead disconnected\n- SMU in compliance\n- SMU Fault = True\rDMM HI SENSE or LO SENSE lead disconnected\n- DMM measures NaN, or \n- DMM overrange warning, or\n- DMM voltage > 50uV "}}, {"Positive Voltage"=nan, "Positive Current"=2.9481971180092548e-05, "Negative Voltage"=nan, "Negative Current"=3.039287802456686e-05, "Impedance"=nan, "ErrorOutData"={"ErrorCode"=-3, "ErrorMessage"="SMU HI or LO lead disconnected\n- SMU in compliance\n- SMU Fault = True\rDMM HI SENSE or LO SENSE lead disconnected\n- DMM measures NaN, or \n- DMM overrange warning, or\n- DMM voltage > 50uV "}}, {"Positive Voltage"=nan, "Positive Current"=2.9481971180092548e-05, "Negative Voltage"=nan, "Negative Current"=3.0267235701188222e-05, "Impedance"=nan, "ErrorOutData"={"ErrorCode"=-3, "ErrorMessage"="SMU HI or LO lead disconnected\n- SMU in compliance\n- SMU Fault = True\rDMM HI SENSE or LO SENSE lead disconnected\n- DMM measures NaN, or \n- DMM overrange warning, or\n- DMM voltage > 50uV "}}, {"Positive Voltage"=nan, "Positive Current"=2.92620971141834e-05, "Negative Voltage"=nan, "Negative Current"=3.03614674437222e-05, "Impedance"=nan, "ErrorOutData"={"ErrorCode"=-3, "ErrorMessage"="SMU HI or LO lead disconnected\n- SMU in compliance\n- SMU Fault = True\rDMM HI SENSE or LO SENSE lead disconnected\n- DMM measures NaN, or \n- DMM overrange warning, or\n- DMM voltage > 50uV "}}, {"Positive Voltage"=nan, "Positive Current"=2.935632885671738e-05, "Negative Voltage"=nan, "Negative Current"=3.039287802456686e-05, "Impedance"=nan, "ErrorOutData"={"ErrorCode"=-3, "ErrorMessage"="SMU HI or LO lead disconnected\n- SMU in compliance\n- SMU Fault = True\rDMM HI SENSE or LO SENSE lead disconnected\n- DMM measures NaN, or \n- DMM overrange warning, or\n- DMM voltage > 50uV "}}, {"Positive Voltage"=nan, "Positive Current"=2.9513381760937207e-05, "Negative Voltage"=nan, "Negative Current"=3.039287802456686e-05, "Impedance"=nan, "ErrorOutData"={"ErrorCode"=-3, "ErrorMessage"="SMU HI or LO lead disconnected\n- SMU in compliance\n- SMU Fault = True\rDMM HI SENSE or LO SENSE lead disconnected\n- DMM measures NaN, or \n- DMM overrange warning, or\n- DMM voltage > 50uV "}}, {"Positive Voltage"=nan, "Positive Current"=2.9576202922623057e-05, "Negative Voltage"=nan, "Negative Current"=3.0267235701188222e-05, "Impedance"=nan, "ErrorOutData"={"ErrorCode"=-3, "ErrorMessage"="SMU HI or LO lead disconnected\n- SMU in compliance\n- SMU Fault = True\rDMM HI SENSE or LO SENSE lead disconnected\n- DMM measures NaN, or \n- DMM overrange warning, or\n- DMM voltage > 50uV "}}, {"Positive Voltage"=nan, "Positive Current"=3.0235825120347032e-05, "Negative Voltage"=nan, "Negative Current"=2.9387739437562038e-05, "Impedance"=nan, "ErrorOutData"={"ErrorCode"=-3, "ErrorMessage"="SMU HI or LO lead disconnected\n- SMU in compliance\n- SMU Fault = True\rDMM HI SENSE or LO SENSE lead disconnected\n- DMM measures NaN, or \n- DMM overrange warning, or\n- DMM voltage > 50uV "}}, {"Positive Voltage"=nan, "Positive Current"=7.078688498982771e-05, "Negative Voltage"=nan, "Negative Current"=-1.1917174372176598e-05, "Impedance"=nan, "ErrorOutData"={"ErrorCode"=-3, "ErrorMessage"="SMU HI or LO lead disconnected\n- SMU in compliance\n- SMU Fault = True\rDMM HI SENSE or LO SENSE lead disconnected\n- DMM measures NaN, or \n- DMM overrange warning, or\n- DMM voltage > 50uV "}}, {"Positive Voltage"=nan, "Positive Current"=4.459046056600954e-05, "Negative Voltage"=nan, "Negative Current"=1.5190156896115886e-05, "Impedance"=nan, "ErrorOutData"={"ErrorCode"=-3, "ErrorMessage"="SMU HI or LO lead disconnected\n- SMU in compliance\n- SMU Fault = True\rDMM HI SENSE or LO SENSE lead disconnected\n- DMM measures NaN, or \n- DMM overrange warning, or\n- DMM voltage > 50uV "}}, {"Positive Voltage"=nan, "Positive Current"=2.929350769502806e-05, "Negative Voltage"=nan, "Negative Current"=3.048710976709737e-05, "Impedance"=nan, "ErrorOutData"={"ErrorCode"=-3, "ErrorMessage"="SMU HI or LO lead disconnected\n- SMU in compliance\n- SMU Fault = True\rDMM HI SENSE or LO SENSE lead disconnected\n- DMM measures NaN, or \n- DMM overrange warning, or\n- DMM voltage > 50uV "}}, {"Positive Voltage"=nan, "Positive Current"=2.923068653334221e-05, "Negative Voltage"=nan, "Negative Current"=2.901081246743306e-05, "Impedance"=nan, "ErrorOutData"={"ErrorCode"=-3, "ErrorMessage"="SMU HI or LO lead disconnected\n- SMU in compliance\n- SMU Fault = True\rDMM HI SENSE or LO SENSE lead disconnected\n- DMM measures NaN, or \n- DMM overrange warning, or\n- DMM voltage > 50uV "}}, {"Positive Voltage"=nan, "Positive Current"=3.290572449207718e-05, "Negative Voltage"=nan, "Negative Current"=2.6906303550892907e-05, "Impedance"=nan, "ErrorOutData"={"ErrorCode"=-3, "ErrorMessage"="SMU HI or LO lead disconnected\n- SMU in compliance\n- SMU Fault = True\rDMM HI SENSE or LO SENSE lead disconnected\n- DMM measures NaN, or \n- DMM overrange warning, or\n- DMM voltage > 50uV "}}, {"Positive Voltage"=nan, "Positive Current"=0.00013326253028835694, "Negative Voltage"=nan, "Negative Current"=-7.150304623306653e-05, "Impedance"=nan, "ErrorOutData"={"ErrorCode"=-3, "ErrorMessage"="SMU HI or LO lead disconnected\n- SMU in compliance\n- SMU Fault = True\rDMM HI SENSE or LO SENSE lead disconnected\n- DMM measures NaN, or \n- DMM overrange warning, or\n- DMM voltage > 50uV "}}, {"Positive Voltage"=nan, "Positive Current"=2.919927595249755e-05, "Negative Voltage"=nan, "Negative Current"=3.0235825120347032e-05, "Impedance"=nan, "ErrorOutData"={"ErrorCode"=-3, "ErrorMessage"="SMU HI or LO lead disconnected\n- SMU in compliance\n- SMU Fault = True\rDMM HI SENSE or LO SENSE lead disconnected\n- DMM measures NaN, or \n- DMM overrange warning, or\n- DMM voltage > 50uV "}}, {"Positive Voltage"=nan, "Positive Current"=2.919927595249755e-05, "Negative Voltage"=nan, "Negative Current"=3.029864628203288e-05, "Impedance"=nan, "ErrorOutData"={"ErrorCode"=-3, "ErrorMessage"="SMU HI or LO lead disconnected\n- SMU in compliance\n- SMU Fault = True\rDMM HI SENSE or LO SENSE lead disconnected\n- DMM measures NaN, or \n- DMM overrange warning, or\n- DMM voltage > 50uV "}}, {"Positive Voltage"=nan, "Positive Current"=2.919927595249755e-05, "Negative Voltage"=nan, "Negative Current"=3.0078772216127203e-05, "Impedance"=nan, "ErrorOutData"={"ErrorCode"=-3, "ErrorMessage"="SMU HI or LO lead disconnected\n- SMU in compliance\n- SMU Fault = True\rDMM HI SENSE or LO SENSE lead disconnected\n- DMM measures NaN, or \n- DMM overrange warning, or\n- DMM voltage > 50uV "}}, {"Positive Voltage"=nan, "Positive Current"=2.8979401886588402e-05, "Negative Voltage"=nan, "Negative Current"=3.0110182796968393e-05, "Impedance"=nan, "ErrorOutData"={"ErrorCode"=-3, "ErrorMessage"="SMU HI or LO lead disconnected\n- SMU in compliance\n- SMU Fault = True\rDMM HI SENSE or LO SENSE lead disconnected\n- DMM measures NaN, or \n- DMM overrange warning, or\n- DMM voltage > 50uV "}}, {"Positive Voltage"=nan, "Positive Current"=2.910504420996704e-05, "Negative Voltage"=nan, "Negative Current"=3.0110182796968393e-05, "Impedance"=nan, "ErrorOutData"={"ErrorCode"=-3, "ErrorMessage"="SMU HI or LO lead disconnected\n- SMU in compliance\n- SMU Fault = True\rDMM HI SENSE or LO SENSE lead disconnected\n- DMM measures NaN, or \n- DMM overrange warning, or\n- DMM voltage > 50uV "}}, {"Positive Voltage"=nan, "Positive Current"=2.913645479080823e-05, "Negative Voltage"=nan, "Negative Current"=3.0204414539502372e-05, "Impedance"=nan, "ErrorOutData"={"ErrorCode"=-3, "ErrorMessage"="SMU HI or LO lead disconnected\n- SMU in compliance\n- SMU Fault = True\rDMM HI SENSE or LO SENSE lead disconnected\n- DMM measures NaN, or \n- DMM overrange warning, or\n- DMM voltage > 50uV "}}, {"Positive Voltage"=nan, "Positive Current"=2.935632885671738e-05, "Negative Voltage"=nan, "Negative Current"=3.0267235701188222e-05, "Impedance"=nan, "ErrorOutData"={"ErrorCode"=-3, "ErrorMessage"="SMU HI or LO lead disconnected\n- SMU in compliance\n- SMU Fault = True\rDMM HI SENSE or LO SENSE lead disconnected\n- DMM measures NaN, or \n- DMM overrange warning, or\n- DMM voltage > 50uV "}}, {"Positive Voltage"=nan, "Positive Current"=2.923068653334221e-05, "Negative Voltage"=nan, "Negative Current"=3.0204414539502372e-05, "Impedance"=nan, "ErrorOutData"={"ErrorCode"=-3, "ErrorMessage"="SMU HI or LO lead disconnected\n- SMU in compliance\n- SMU Fault = True\rDMM HI SENSE or LO SENSE lead disconnected\n- DMM measures NaN, or \n- DMM overrange warning, or\n- DMM voltage > 50uV "}}, {"Positive Voltage"=nan, "Positive Current"=2.92620971141834e-05, "Negative Voltage"=nan, "Negative Current"=3.0141593377813053e-05, "Impedance"=nan, "ErrorOutData"={"ErrorCode"=-3, "ErrorMessage"="SMU HI or LO lead disconnected\n- SMU in compliance\n- SMU Fault = True\rDMM HI SENSE or LO SENSE lead disconnected\n- DMM measures NaN, or \n- DMM overrange warning, or\n- DMM voltage > 50uV "}}, {"Positive Voltage"=nan, "Positive Current"=2.919927595249755e-05, "Negative Voltage"=nan, "Negative Current"=3.0110182796968393e-05, "Impedance"=nan, "ErrorOutData"={"ErrorCode"=-3, "ErrorMessage"="SMU HI or LO lead disconnected\n- SMU in compliance\n- SMU Fault = True\rDMM HI SENSE or LO SENSE lead disconnected\n- DMM measures NaN, or \n- DMM overrange warning, or\n- DMM voltage > 50uV "}}, {"Positive Voltage"=nan, "Positive Current"=2.901081246743306e-05, "Negative Voltage"=nan, "Negative Current"=3.0204414539502372e-05, "Impedance"=nan, "ErrorOutData"={"ErrorCode"=-3, "ErrorMessage"="SMU HI or LO lead disconnected\n- SMU in compliance\n- SMU Fault = True\rDMM HI SENSE or LO SENSE lead disconnected\n- DMM measures NaN, or \n- DMM overrange warning, or\n- DMM voltage > 50uV "}}, {"Positive Voltage"=nan, "Positive Current"=2.913645479080823e-05, "Negative Voltage"=nan, "Negative Current"=3.0078772216127203e-05, "Impedance"=nan, "ErrorOutData"={"ErrorCode"=-3, "ErrorMessage"="SMU HI or LO lead disconnected\n- SMU in compliance\n- SMU Fault = True\rDMM HI SENSE or LO SENSE lead disconnected\n- DMM measures NaN, or \n- DMM overrange warning, or\n- DMM voltage > 50uV "}}, {"Positive Voltage"=nan, "Positive Current"=2.913645479080823e-05, "Negative Voltage"=nan, "Negative Current"=3.0173003958657713e-05, "Impedance"=nan, "ErrorOutData"={"ErrorCode"=-3, "ErrorMessage"="SMU HI or LO lead disconnected\n- SMU in compliance\n- SMU Fault = True\rDMM HI SENSE or LO SENSE lead disconnected\n- DMM measures NaN, or \n- DMM overrange warning, or\n- DMM voltage > 50uV "}}]
  in  "Default Results":T2[](array[typedef])
  out "Channel Index":i32=160
  out "Result":T2={"Positive Voltage"=nan, "Positive Current"=2.913645479080823e-05, "Negative Voltage"=nan, "Negative Current"=3.0078772216127203e-05, "Impedance"=nan, "ErrorOutData"={"ErrorCode"=-3, "ErrorMessage"="SMU HI or LO lead disconnected\n- SMU in compliance\n- SMU Fault = True\rDMM HI SENSE or LO SENSE lead disconnected\n- DMM measures NaN, or \n- DMM overrange warning, or\n- DMM voltage > 50uV "}}
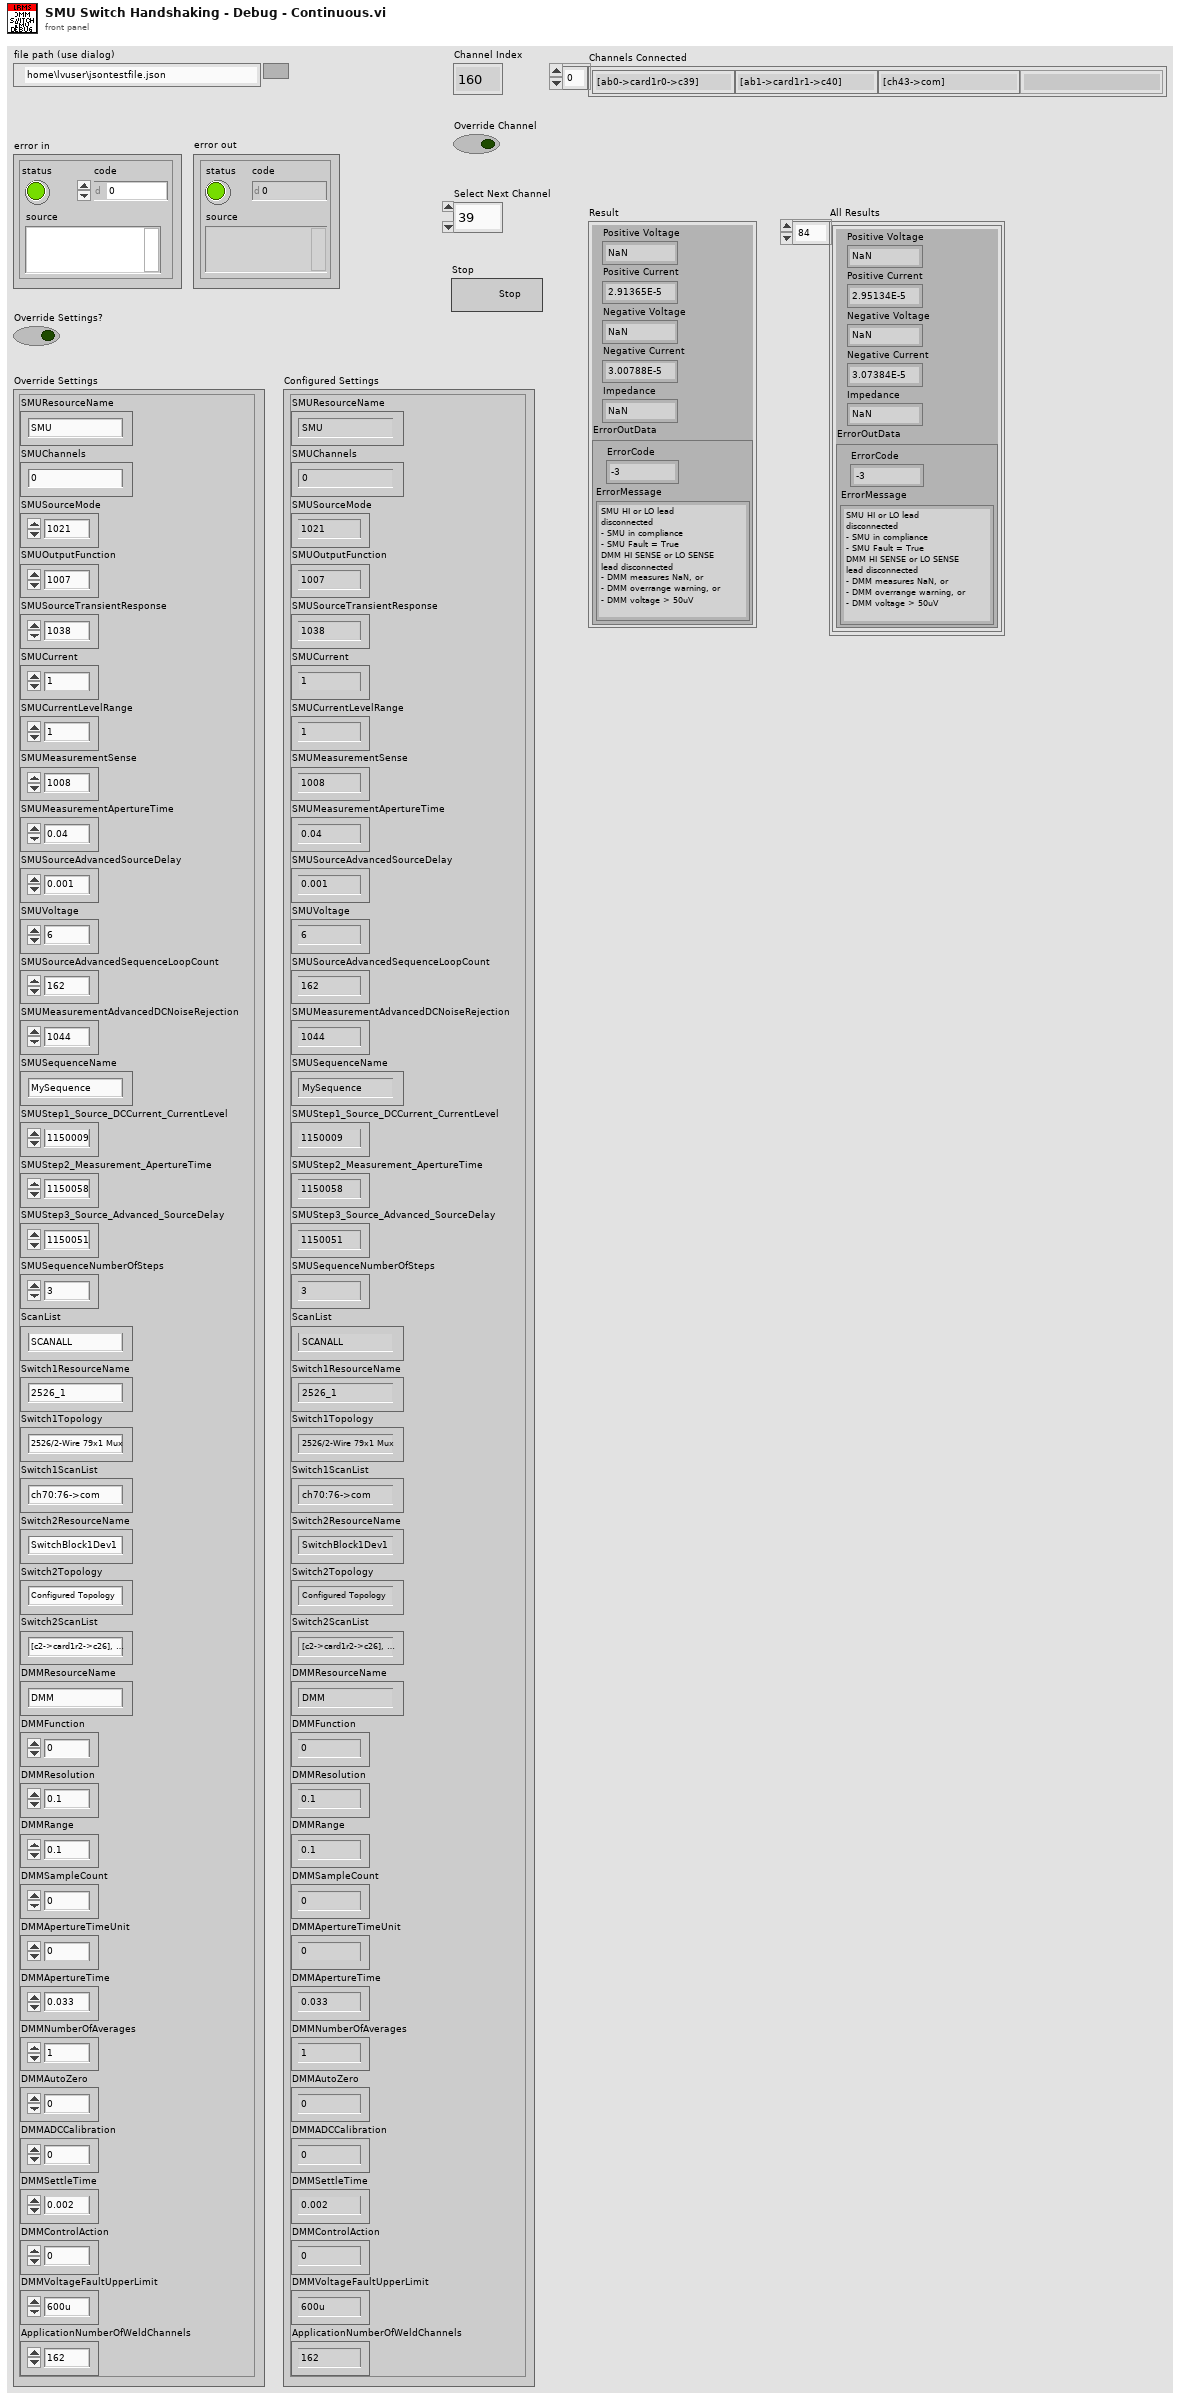
[diagram p1: front panel]
types:
  T1 = typedef "JSONCluster.ctl" = cluster{"SMUResourceName":string, "SMUChannels":string, "SMUSourceMode":i32, "SMUOutputFunction":i32, "SMUSourceTransientResponse":i32, "SMUCurrent":dbl, "SMUCurrentLevelRange":dbl, "SMUMeasurementSense":i32, "SMUMeasurementApertureTime":dbl, "SMUSourceAdvancedSourceDelay":dbl, "SMUVoltage":dbl, "SMUSourceAdvancedSequenceLoopCount":i32, "SMUMeasurementAdvancedDCNoiseRejection":i32, "SMUSequenceName":string, "SMUStep1_Source_DCCurrent_CurrentLevel":i32, "SMUStep2_Measurement_ApertureTime":i32, "SMUStep3_Source_Advanced_SourceDelay":i32, "SMUSequenceNumberOfSteps":i32, "ScanList":string, "Switch1ResourceName":string, "Switch1Topology":string, "Switch1ScanList":string, "Switch2ResourceName":string, "Switch2Topology":string, "Switch2ScanList":string, "DMMResourceName":string, "DMMFunction":i32, "DMMResolution":dbl, "DMMRange":dbl, "DMMSampleCount":i32, "DMMApertureTimeUnit":i32, "DMMApertureTime":dbl, "DMMNumberOfAverages":i32, "DMMAutoZero":i32, "DMMADCCalibration":i32, "DMMSettleTime":dbl, "DMMControlAction":i32, "DMMVoltageFaultUpperLimit":dbl, "ApplicationNumberOfWeldChannels":i32}
  T2 = typedef "labview-grpc-measurement-server.lvlib/MeasurementServer_FourProbeRawData.ctl" = cluster{"Positive Voltage":dbl, "Positive Current":dbl, "Negative Voltage":dbl, "Negative Current":dbl, "Impedance":dbl, "ErrorOutData":T3}
  T3 = typedef "labview-grpc-measurement-server.lvlib/MeasurementServer_ErrorOutData.ctl" = cluster{"ErrorCode":i32, "ErrorMessage":string}
  T4 = typedef "niDCPower Send Software Edge Trigger - Signal.ctl" = i32
  T5 = typedef "niDMM Acquisition State.ctl" = enum16{"Running", "Finished with Backlog", "Finished with no Backlog", "Paused", "No acquisition in progress"}
  T6 = typedef "niDCPower Wait For Event - Event.ctl" = i32
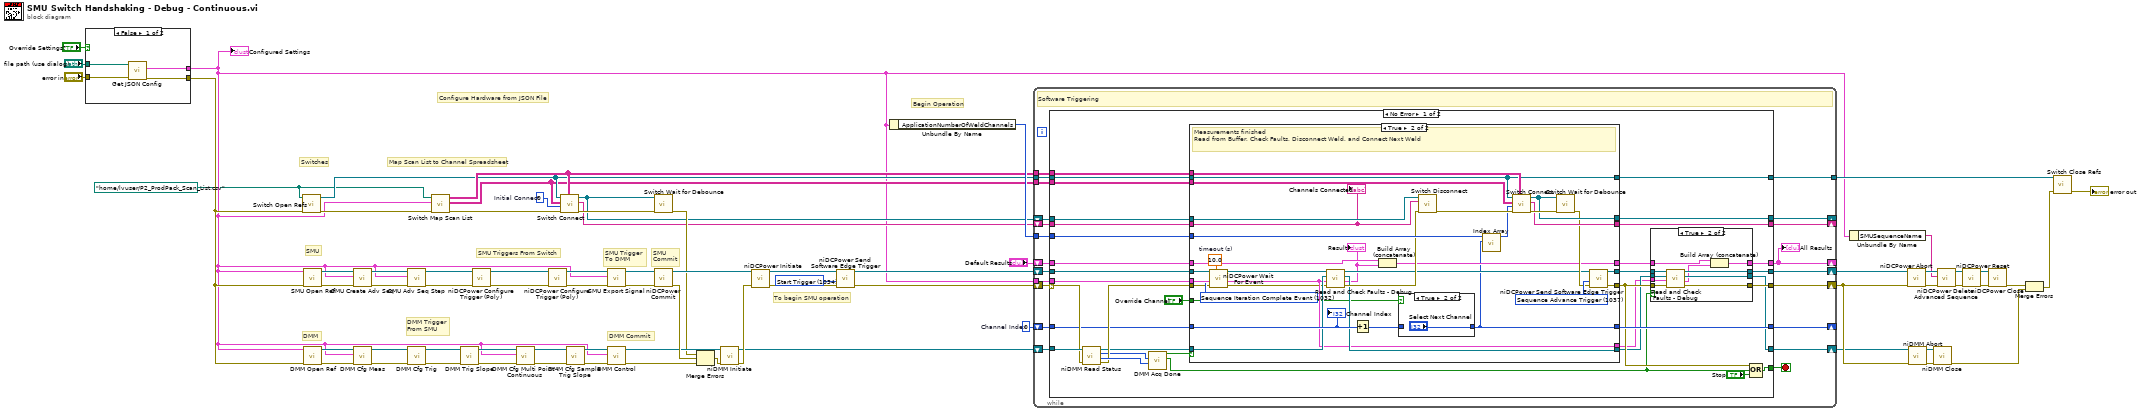
[diagram p0: block diagram]
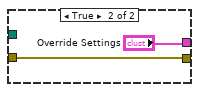
[diagram p2: hidden frame]
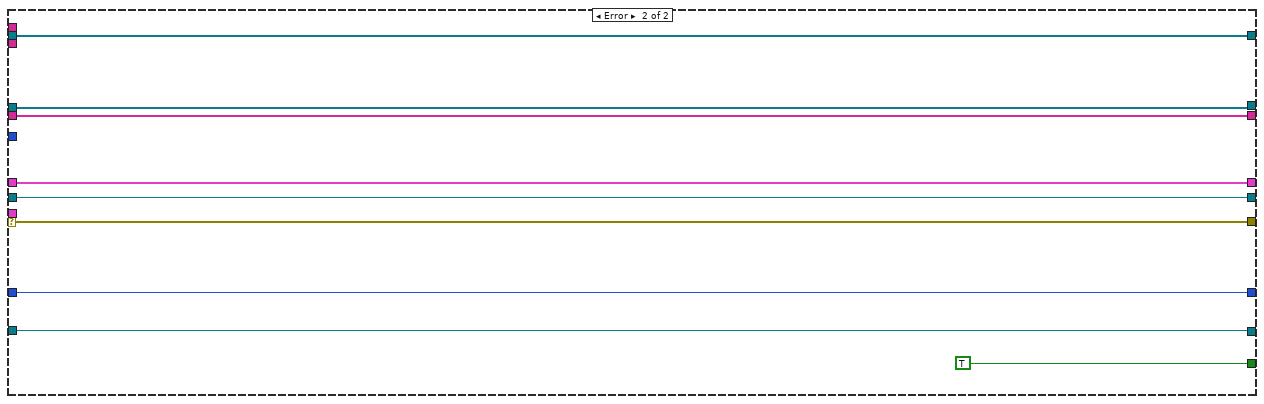
[diagram p6: hidden frame]
diagram:
  w1 = path "/home/lvuser/P2_ProdPack_Scan_List.csv" ("Ch Spreadsheet")
  w17 = 0  # Initial Connect
  w29 = 0  # Channel Index
  w30 = T4 1034 items=["Start Trigger"=1034, "Source Trigger"=1035, "Measure Trigger"=1036, "Sequence Advance Trigger"=1037, "Pulse Trigger"=1053] ("signal")
  # "Map Scan List to Channel Spreadsheet"
  # "SMU\nCommit"
  # "DMM Commit"
  # "Begin Operation"
  # "Configure Hardware from JSON File"
  # "DMM"
  # "SMU"
  # "Switches"
  # "To begin SMU operation"
  # "DMM Trigger\nFrom SMU"
  # "SMU Trigger \nTo DMM"
  # "SMU Triggers From Switch"
  n1 = case shown="False" "Override Settings?" {
    tunnel: "file path (use dialog)" -> [w76 _]
    tunnel: "error in" -> [w75 w78]
    tunnel: [w74 w78] -> w16
    tunnel: [w73 "Override Settings"] -> w6
    frame False {
      n2 = call "Get JSON Config.vi"("error in (no error)"=w75, "JSON Configuration File (.json)"=w76) -> ("error out"=w74:errorcluster, "JSONCluster"=w73:T1)  [unwired: 6 in, 2 out]
    }
    frame True {
    }
  }
  "Configured Settings" <- w6
  n3 = call "Switch Open Refs.vi"("error in"=w16, "CSV File"=w1) -> ("error out"=w20:errorcluster, "Switch Refs"=w13:refnum<k15>[])  [unwired: 8 in]
  n4 = call "SMU Open Ref.vi"("error in (no error)"=w16, "JSONCluster"=w6) -> ("error out"=w71:errorcluster, "IVI Refnum out"=w72:refnum<k15>)  [unwired: 8 in]
  n5 = call "DMM Open Ref.vi"("error in"=w16, "JSONCluster"=w6) -> ("error out"=w46:errorcluster, "IVI Refnum out"=w45:refnum<k15>)  [unwired: 8 in]
  n6 = call "SMU Create Adv Seq.vi"("error in (no error)"=w71, "JSONCluster"=w6, "IVI Refnum in"=w72) -> ("error out"=w61:errorcluster, "IVI Refnum out"=w62:refnum<k15>)  [unwired: 7 in]
  n7 = call "DMM Cfg Meas.vi"("error in (no error)"=w46, "JSONCluster"=w6, "IVI Refnum in"=w45) -> ("error out"=w50:errorcluster, "IVI Refnum out"=w49:refnum<k15>)  [unwired: 7 in]
  n8 = call "SMU Adv Seq Step.vi"("error in (no error)"=w61, "JSONCluster"=w6, "IVI Refnum in"=w62) -> ("error out"=w59:errorcluster, "IVI Refnum out"=w60:refnum<k15>)  [unwired: 7 in]
  n9 = call "DMM Cfg Trig.vi"("error in (no error)"=w50, "IVI Refnum in"=w49) -> ("error out"=w52:errorcluster, "IVI Refnum out"=w51:refnum<k15>)  [unwired: 8 in]
  n10 = call "Switch Map Scan List.vi"("error in (no error)"=w20, "JSONCluster"=w6, "Ch Spreadsheet"=w1) -> ("error out"=w19:errorcluster, "IVI Specifications"=w12:string[][], "Channel Specs"=w14:string[][])  [unwired: 6 in]
  n11 = call "DMM Trig Slope.vi"("error in (no error)"=w52, "IVI Refnum in"=w51) -> ("error out"=w54:errorcluster, "IVI Refnum out"=w53:refnum<k15>)  [unwired: 8 in]
  n12 = call-poly <instrlib>:"niDCPower Configure Trigger (Poly).vi"("error in (no error)"=w59, "instrument handle"=w60) -> ("error out"=w69:errorcluster, "instrument handle out"=w70:refnum<k15>)  [unwired: 8 in]
  n13 = call "DMM Cfg Multi Point - Continuous.vi"("error in (no error)"=w54, "JSONCluster"=w6, "IVI Refnum in"=w53) -> ("error out"=w56:errorcluster, "IVI Refnum out"=w55:refnum<k15>)  [unwired: 7 in]
  n14 = call-poly <instrlib>:"niDCPower Configure Trigger (Poly).vi"("error in (no error)"=w69, "instrument handle"=w70) -> ("error out"=w34:errorcluster, "instrument handle out"=w35:refnum<k15>)  [unwired: 8 in]
  n15 = call "Switch Connect.vi"("Channel Specs"=w14, "error in (no error)"=w19, "Channel Index"=w17, "IVI Specifications"=w12, "Switch Refs"=w13) -> ("error out"=w18:errorcluster, "Channels Connected"=w10:string[], "Refs Connected"=w11:refnum<k15>[])  [unwired: 4 in]
  n16 = call "DMM Cfg Sample Trig Slope.vi"("error in (no error)"=w56, "IVI Refnum in"=w55) -> ("error out"=w38:errorcluster, "IVI Refnum out"=w39:refnum<k15>)  [unwired: 8 in]
  n17 = call "SMU Export Signal.vi"("error in (no error)"=w34, "JSONCluster"=w6, "IVI Refnum in"=w35) -> ("error out"=w57:errorcluster, "IVI Refnum out"=w58:refnum<k15>)  [unwired: 7 in]
  n18 = call "DMM Control.vi"("error in (no error)"=w38, "JSONCluster"=w6, "IVI Refnum in"=w39) -> ("error out"=w43:errorcluster, "IVI Refnum out"=w40:refnum<k15>)  [unwired: 7 in]
  n19 = call "Switch Wait for Debounce.vi"("error in (no error)"=w18, "Switch Refs"=w11) -> ("error out"=w15:errorcluster)  [unwired: 9 in]
  n20 = call <instrlib>:"niDCPower Commit.vi"("error in (no error)"=w57, "instrument handle"=w58) -> ("error out"=w44:errorcluster, "instrument handle out"=w41:refnum<k15>)  [unwired: 8 in]
  n21 = Merge Errors(w15, w44, w43) -> (w42:errorcluster)
  n22 = call <instrlib>:"niDMM Initiate.vi"("error in (no error)"=w42, "instrument handle"=w40) -> ("error out"=w26:errorcluster, "instrument handle out"=w23:refnum<k15>)  [unwired: 8 in]
  n23 = call <instrlib>:"niDCPower Initiate.vi"("error in (no error)"=w26, "instrument handle"=w41) -> ("error out"=w27:errorcluster, "instrument handle out"=w31:refnum<k15>)  [unwired: 8 in]
  n24 = call <instrlib>:"niDCPower Send Software Edge Trigger.vi"("error in (no error)"=w27, "signal"=w30, "instrument handle"=w31) -> ("error out"=w21:errorcluster, "instrument handle out"=w24:refnum<k15>)  [unwired: 7 in]
  n25 = Unbundle By Name(w6) -> ("ApplicationNumberOfWeldChannels"=w28:i32)
  n26 = while {
    shift-right: [w99] -> w5
    shift-left: w24 -> [w98]
    shift-right: [w92] -> w22
    shift-left: w21 -> [w90]
    shift-right: [w94] -> w4
    shift-left: w23 -> [w95]
    shift-right: [w97] -> _
    shift-left: w29 -> [w93]
    tunnel: w28 -> [w96]
    tunnel: w14 -> [w89]
    tunnel: w13 -> [w88]
    tunnel: w12 -> [w87]
    shift-right: [w83] -> _
    shift-left: w11 -> [w86]
    shift-right: [w82] -> _
    shift-left: w10 -> [w85]
    tunnel: [w84] -> w9
    tunnel: w6 -> [w81]
    shift-right: [w79] -> _
    shift-left: "Default Results" -> [w80]
    stop <- w91 stop-if-true
    # "Software Triggering"
    n27 = case shown="No Error" w90 {
      selector: w90 -> [w126 w197]
      tunnel: [w106 w196] -> w99
      tunnel: w98 -> [w133 w196]
      tunnel: [w132 w198] -> w97
      tunnel: w96 -> [w131 _]
      tunnel: w95 -> [w129 w199]
      tunnel: [w104 w199] -> w94
      tunnel: w93 -> [w125 w198]
      tunnel: [w111 w197] -> w92
      tunnel: [w124 TRUE] -> w91
      tunnel: w89 -> [w123 _]
      tunnel: w88 -> [w122 w195]
      tunnel: w87 -> [w121 _]
      tunnel: w86 -> [w120 w194]
      tunnel: w85 -> [w119 w193]
      tunnel: [w118 w195] -> w84
      tunnel: [w117 w194] -> w83
      tunnel: [w116 w193] -> w82
      tunnel: w81 -> [w114 _]
      tunnel: w80 -> [w113 w192]
      tunnel: [w109 w192] -> w79
      frame No Error {
        n28 = call <instrlib>:"niDMM Read Status.vi"("error in (no error)"=w126, "instrument handle"=w129) -> ("error out"=w128:errorcluster, "Acquisition State"=w130:T5, "Backlog"=w100:i32, "instrument handle out"=w115:refnum<k15>)  [unwired: 6 in]
        n29 = call "DMM Acq Done.vi"("Acquisition State"=w130, "Backlog"=w100) -> ("Finished with Backlog?"=w108:bool, "Sequence Acquision Finished?"=w127:bool)  [unwired: 8 in]
        n30 = case shown="True" w127 {
          tunnel: w128 -> [w155 w159]
          tunnel: [w156 w189] -> w107
          tunnel: [w155 w188] -> w112
          tunnel: w133 -> [w156 w160]
          tunnel: w125 -> [w154 w186]
          tunnel: [w154 w164] -> w132
          tunnel: w131 -> [_ w185]
          tunnel: w123 -> [_ w182]
          tunnel: w122 -> [w153 w177]
          tunnel: w121 -> [_ w181]
          tunnel: w120 -> [w152 w180]
          tunnel: w119 -> [w151 w179]
          tunnel: [w153 w177] -> w118
          tunnel: [w152 w176] -> w117
          tunnel: [w151 w175] -> w116
          tunnel: w115 -> [w150 w171]
          tunnel: [w150 w170] -> w105
          tunnel: w114 -> [w148 w168]
          tunnel: w113 -> [w149 w167]
          tunnel: [w149 w169] -> w110
          tunnel: [w148 w168] -> w103
          tunnel: "Override Channel" -> [_ w163]
          frame False {
            # "Measurements not finished yet - repeat loop"
          }
          frame True {
            w161 = 10.0  # timeout (s)
            w162 = T6 1032 items=["Source Complete Event"=1030, "Measure Complete Event"=1031, "Sequence Iteration Complete Event"=1032, "Sequence Engine Done Event"=1033, "Pulse Complete Event"=1051, "Ready For Pulse Trigger Event"=1052] ("event")
            w187 = T4 1037 items=["Start Trigger"=1034, "Source Trigger"=1035, "Measure Trigger"=1036, "Sequence Advance Trigger"=1037, "Pulse Trigger"=1053] ("signal")
            # "Measurements finished\nRead from Buffer, Check Faults, Disconnect Weld, and Connect Next Weld"
            n31 = call <instrlib>:"niDCPower Wait For Event.vi"("timeout (sec)"=w161, "error in (no error)"=w159, "event"=w162, "instrument handle"=w160) -> ("error out"=w157:errorcluster, "instrument handle out"=w158:refnum<k15>)  [unwired: 6 in]
            n32 = call "Read and Check Faults - Debug.vi"("error in (no error)"=w157, "JSONCluster"=w168, "DMM Ref"=w171, "SMU Ref"=w158) -> ("error out"=w173:errorcluster, "Result"=w166:T2, "DMM Ref Out"=w170:refnum<k15>, "SMU Ref Out"=w172:refnum<k15>)  [unwired: 4 in]
            "Result" <- w166
            n33 = Increment(x=w186) -> (x+1=w165:i32)
            n34 = Build Array (concatenate)(w167, w166) -> (w169:T2[])
            n35 = case shown="True" w163 {
              tunnel: w165 -> [w190 _]
              tunnel: [w190 "Select Next Channel"] -> w164
              frame False {
              }
              frame True {
              }
            }
            n36 = call "Switch Disconnect.vi"("error in (no error)"=w173, "Channels Connected"=w179, "Switch Refs"=w180) -> ("error out"=w184:errorcluster)  [unwired: 8 in]
            n37 = call "Index Array.vi"("Backlog"=w164, "ApplicationNumberOfWeldChannels"=w185) -> ("Index"=w178:i32)  [unwired: 9 in]
            n38 = call "Switch Connect.vi"("Channel Specs"=w182, "error in (no error)"=w184, "Channel Index"=w178, "IVI Specifications"=w181, "Switch Refs"=w177) -> ("error out"=w183:errorcluster, "Channels Connected"=w175:string[], "Refs Connected"=w176:refnum<k15>[])  [unwired: 4 in]
            n39 = call "Switch Wait for Debounce.vi"("error in (no error)"=w183, "Switch Refs"=w176) -> ("error out"=w174:errorcluster)  [unwired: 9 in]
            n40 = call <instrlib>:"niDCPower Send Software Edge Trigger.vi"("error in (no error)"=w174, "signal"=w187, "instrument handle"=w172) -> ("error out"=w188:errorcluster, "instrument handle out"=w189:refnum<k15>)  [unwired: 7 in]
            "Channel Index" <- w186
            "Channels Connected" <- w179
          }
        }
        n41 = case shown="True" w108 {
          tunnel: w112 -> [w135 w147]
          tunnel: [w135 w146] -> w111
          tunnel: w110 -> [w137 w139]
          tunnel: [w137 w145] -> w109
          tunnel: w107 -> [w136 w144]
          tunnel: [w136 w143] -> w106
          tunnel: w105 -> [w134 w142]
          tunnel: [w134 w141] -> w104
          tunnel: w103 -> [_ w140]
          frame False {
          }
          frame True {
            n42 = call "Read and Check Faults - Debug.vi"("error in (no error)"=w147, "JSONCluster"=w140, "DMM Ref"=w142, "SMU Ref"=w144) -> ("error out"=w146:errorcluster, "Result"=w138:T2, "DMM Ref Out"=w141:refnum<k15>, "SMU Ref Out"=w143:refnum<k15>)  [unwired: 4 in]
            n43 = Build Array (concatenate)(w139, w138) -> (w145:T2[])
          }
        }
        n44 = Compound Arithmetic op=OR(w112, w108, "Stop") -> (w124:bool)
      }
      frame Error {
      }
    }
    "All Results" <- w79
  }
  n45 = Unbundle By Name(w6) -> ("SMUSequenceName"=w25:string)
  n46 = call <instrlib>:"niDCPower Abort.vi"("error in (no error)"=w22, "instrument handle"=w5) -> ("error out"=w67:errorcluster, "instrument handle out"=w68:refnum<k15>)  [unwired: 8 in]
  n47 = call <instrlib>:"niDMM Abort.vi"("error in (no error)"=w22, "instrument handle"=w4) -> ("error out"=w48:errorcluster, "instrument handle out"=w47:refnum<k15>)  [unwired: 8 in]
  n48 = call <instrlib>:"niDMM Close.vi"("error in (no error)"=w48, "instrument handle"=w47) -> ("error out"=w37:errorcluster)  [unwired: 9 in]
  n49 = call <instrlib>:"niDCPower Delete Advanced Sequence.vi"("error in (no error)"=w67, "sequence name"=w25, "instrument handle"=w68) -> ("error out"=w66:errorcluster, "instrument handle out"=w65:refnum<k15>)  [unwired: 7 in]
  n50 = call <instrlib>:"niDCPower Reset.vi"("error in (no error)"=w66, "instrument handle"=w65) -> ("error out"=w63:errorcluster, "instrument handle out"=w64:refnum<k15>)  [unwired: 2 in, 6 out]
  n51 = call <instrlib>:"niDCPower Close.vi"("error in (no error)"=w63, "instrument handle"=w64) -> ("error out"=w36:errorcluster)  [unwired: 9 in]
  n52 = Merge Errors(w36, w37) -> (w8:errorcluster)
  n53 = call "Switch Close Refs.vi"("error in (no error)"=w8, "Switch Refs"=w9) -> ("error out"=→"error out":errorcluster)  [unwired: 9 in]
